vi "GUMSSequenceGeneratorV3.vi"() -> ()   [LabVIEW 2011]
uses:
  Kelvinox drivers/ITCAPPS - Copie.LLB/ITCSignal.ctl
  Kelvinox drivers/ITCAPPS.LLB/ITCSignals.ctl
  DAC/Visa name1.vi
  GlobalVar.vi
  stopButton.vi
  monochromatorcontrol/perHandlemonochromator.vi
  monochromatorcontrol/libPhyspec.lvlib
panel:
  out "loopchange 2":u32
  out "LockinX":string[][](array[string])
  in  "Device Cluster":T3={"K2400 1"="", "K2400_1"=FALSE, "K2400 2"="", "K2400_2"=FALSE, "TIC"="", "Tcontrol"="OFF", "DAC"="", "DAC present"=FALSE, "Bfield query"=FALSE, "Wvlen query"=FALSE, "ITC signal"={"ITC"=0, "Signal"=enum."Sensor 1"}, "DMMX"=[["DMM1", ""]], "LockinX"=[["DMM1", ""]]}
  in  "Gain Cluster":T4={"Vsd"="Gate", "I 2probe"="Gate", "Vxy"="Gate", "Vxx"="Gate", "I leak BG"="Gate", "I leak TG"="Gate", "I Gain 1"=1000000.0, "V Gain 1"=1.0, "conversion factor BG"=1.0, "Vin / Vout 1"=1.0, "V Gain 2"=1.0, "Vin / Vout 2"=1.0, "V Gain 3"=1.0, "Vin / Vout 3"=1.0, "I Gain 2"=1000000.0, "I Gain 3"=1000000.0, "V BG"="Gate", "V TG"="Gate", "conversion factor TG"=1.0, "Vin / Vout 4"=1.0, "Vin / Vout 5"=1.0, "Manual Gain 1"=1.0, "Manual Gain 2"=1.0, "Manual Gain 3"=1.0, "V / I 4"="Gate", "V / I 3"="Gate", "Gain V/I3"=1.0, "Gain V/I4"=1.0} {"conversion factor TG" items=["1 V/V"=1.0, "4 V/V"=4.0, "15 V/V"=15.0, "30 V/V"=30.0, "45 V/V"=45.0]; "I Gain 3" items=["1"=1.0, "10"=10.0, "100"=100.0, "1K"=1000.0, "10K"=10000.0, "100K"=100000.0, "1M"=1000000.0, "10M"=10000000.0, "100M"=100000000.0, "1G"=1000000000.0]; "I Gain 2" items=["1"=1.0, "10"=10.0, "100"=100.0, "1K"=1000.0, "10K"=10000.0, "100K"=100000.0, "1M"=1000000.0, "10M"=10000000.0, "100M"=100000000.0, "1G"=1000000000.0]; "V Gain 3" items=["1"=1.0, "10"=10.0, "100"=100.0, "1K"=1000.0, "10K"=10000.0]; "V Gain 2" items=["1"=1.0, "10"=10.0, "100"=100.0, "1K"=1000.0, "10K"=10000.0]; "conversion factor BG" items=["1 V/V"=1.0, "4 V/V"=4.0, "15 V/V"=15.0, "30 V/V"=30.0, "45 V/V"=45.0]; "V Gain 1" items=["1"=1.0, "10"=10.0, "100"=100.0, "1K"=1000.0, "10K"=10000.0]; "I Gain 1" items=["1"=1.0, "10"=10.0, "100"=100.0, "1K"=1000.0, "10K"=10000.0, "100K"=100000.0, "1M"=1000000.0, "10M"=10000000.0, "100M"=100000000.0, "1G"=1000000000.0]}
  out "counter 2":i32
  out "DMMX":string[][](array[string])
  out "Bloop gen":u32
  out "WVlenloop gen":u32
  out "Tloop gen":u32
  out "loopchange":u32
  out "DACindic":bool
  in  "EmptyAllArrays":bool
  in  "Sweep back to zero":bool
  out "counter":i32
  out "Num elements in col":i32[](array[numeric])
  out "Current col":i32
  in  "Refresh Rate [ms]":i32=1000 min=0
  out "Current sweep":dbl
  out "ITC ref":T1={"ITC"=0, "Signal"=enum."Sensor 3"}
  in  "Cancel run":bool
  out "DAC":refnum<visa-resource-name>
  out "K2400 2":refnum<visa-resource-name>
  out "Lockin1":refnum<visa-resource-name>
  out "K2400 1":refnum<visa-resource-name>
  out "Total sweep sequence":dbl[][](array[numeric])
  in  "Tab Control":T5(tab)
  in  "Sweep Toothsaw":bool
  in  "Loop Cluster":T6
  in  "START":bool
  in  "genTotalSequence":bool
  out "row state":i32[](array[numeric])
  out "Priority type array":string[](array[string])
  out "TotalPnts":dbl
  in  "Sweep back\nto zero?":bool
  in  "Conversion Factor Fix\n1 V = ??":dbl=1.0
  in  "Fix type":string(combo)
  in  "Sweep Bias":dbl[](array[numeric])
  in  "Fix Bias":dbl[](array[numeric])
  in  "Priority sweep":i32=2
  in  "Priority fix":i32=2
  in  "sweep start [V]":dbl=-1.0 min=-200.0 max=200.0
  in  "sweep stop [V]":dbl=-5.0 min=-250.0 max=250.0
  in  "Nb steps":i32=800
  in  "sweep stop 2 [V]":dbl min=-250.0 max=250.0
  in  "Nb steps 2":i32
  in  "Nb Sweep":i32=1
  in  "Nb steps fix2":i32
  in  "Fix stop 2":dbl min=-250.0 max=250.0
  in  "Nb steps fix":i32=800
  in  "Fix stop":dbl=-5.0 min=-250.0 max=250.0
  in  "Fix start":dbl=-1.0 min=-200.0 max=200.0
  in  "genSweepArray":bool
  in  "genFixArray":bool
  in  "Sweep Instrument":string(combo)
  in  "Conversion Factor Sweep\n1 V = ??":dbl=1.0
  in  "Fix Instrument":string(combo)
  in  "Sweep type":string(combo)
  in  "V step K2400 [V]":dbl=0.001
  in  "genSweepArray sweeploop":bool
  in  "genfixArray fixlooop simple":bool
  in  "Nb steps VI4 2":i32
  in  "VI4 stop2":dbl min=-250.0 max=250.0
  in  "Nb steps VI4":i32=800
  in  "VI4 stop1":dbl=-5.0 min=-250.0 max=250.0
  in  "genVI4Array":bool
  in  "genVI4Array simple":bool
  in  "Increase neg":dbl
  in  "Steps neg":dbl
  in  "Sweeps":i32
  in  "Steps 2":dbl
  in  "Bgstop 2":dbl
  in  "Steps":dbl
  in  "Bgstop":dbl
  in  "IOL ramp":dbl[](array[numeric])
  in  "VI 4 Array":dbl[](array[numeric])
  in  "Bgstart":dbl
  in  "Loops":i32
  in  "Increase pos":dbl
  in  "Steps pos":dbl
  in  "genIonicRamp":bool
  in  "Conversion Factor IOL Ramp\n1 V = ??":dbl=1.0
  in  "Conversion Factor VI4\n1 V = ??":dbl=1.0
  in  "VI4 start (V or I)":dbl=-1.0 min=-200.0 max=200.0
  in  "Stabilization Time (s)":i32 min=-200 max=200
  in  "T Rate [K/min]":dbl min=-200.0 max=200.0
  in  "T [K]":dbl[](array[numeric])
  in  "Priority T":i32=2
  in  "Nb T steps":i32=800
  in  "T stop [K]":dbl=-1.0 min=-200.0 max=200.0
  in  "T start [K]":dbl=-1.0 min=-200.0 max=200.0
  in  "genTarray":bool
  in  "Add T points":bool
  in  "Zero ramp Rate [T/min] 2":dbl=0.2 min=-200.0 max=200.0
  in  "Sweep Field back to zero":bool
  in  "B [T]":dbl[](array[numeric])
  in  "B start [T]":dbl=-1.0 min=-200.0 max=200.0
  in  "B stop [T]":dbl=-1.0 min=-200.0 max=200.0
  in  "Sweep Rate [T/min]":dbl=0.1 min=-200.0 max=200.0
  in  "Nb B steps":i32=800
  in  "GenBarray":bool
  in  "Add B points":bool
  in  "Set Persistent":bool=TRUE
  in  "PEM retardation (lambda)":dbl=1.0 min=0.0 max=1.0
  in  "PEM present ?":bool=TRUE
  in  "Power stabilization":bool=TRUE
  in  "Wvlen Start [nm]":dbl=400.0
  in  "Wavelength [nm]":dbl[](array[numeric])
  in  "genWVLEN array":bool
  in  "Add wvlen points":bool
  in  "Nb Wvlen steps":i32=350
  in  "Wvlen stop [nm]":dbl=1100.0
  out "Laser Power [W]":dbl format="%#.2g"
  in  "PEM VISA":refnum<visa-resource-name>
  in  "START FC":bool
  out "Field ok !":bool
  in  "Bipolar":bool
  in  "High T (K)":dbl
  in  "Temperature Up rate (K/min)":dbl
  in  "Waiting time (min)":dbl
  in  "Base T (K)":dbl
  in  "sweep rate B (T/min)":dbl
  in  "Cooling field (T)":dbl
  out "I am":string
  in  "File Basename":string
  out "Bias factor":dbl
  in  "Nb steps Increase 2":dbl=10.0
  in  "Gate Increase 2 (V)":dbl=0.1
  in  "Nb steps Increase":dbl=10.0
  in  "Gate Increase (V)":dbl=-0.1
  out "x .or. y?":bool
  in  "Step Delay (ms)":dbl=1000.0
  out "Total Progress":dbl(slide) scale=0.0..1.0
  in  "Nb Loop":i32
  out "Nb Loop Indicator":i32=2
  out "Nb Sweep Indicator":i32=3
  out "conversion factor sweep":dbl(ring)=1.0 items=["1 V/V"=1.0, "4 V/V"=4.0, "15 V/V"=15.0, "30 V/V"=30.0, "45 V/V"=45.0]
  in  "stop":bool
  in  "V step [V]":dbl=0.001
  in  "Folder Name":path=path "D:/users/marc/20180122_LiIon_EL/Freezing02/OutputHighT002p2.dat"
  # "Magnetic Field"
  # "Wavelength"
  # "IV Sweep Setting"
  # "IV Fix Setting"
  # "Ionic Liquid Ramp"
  # "VI 4 Array"
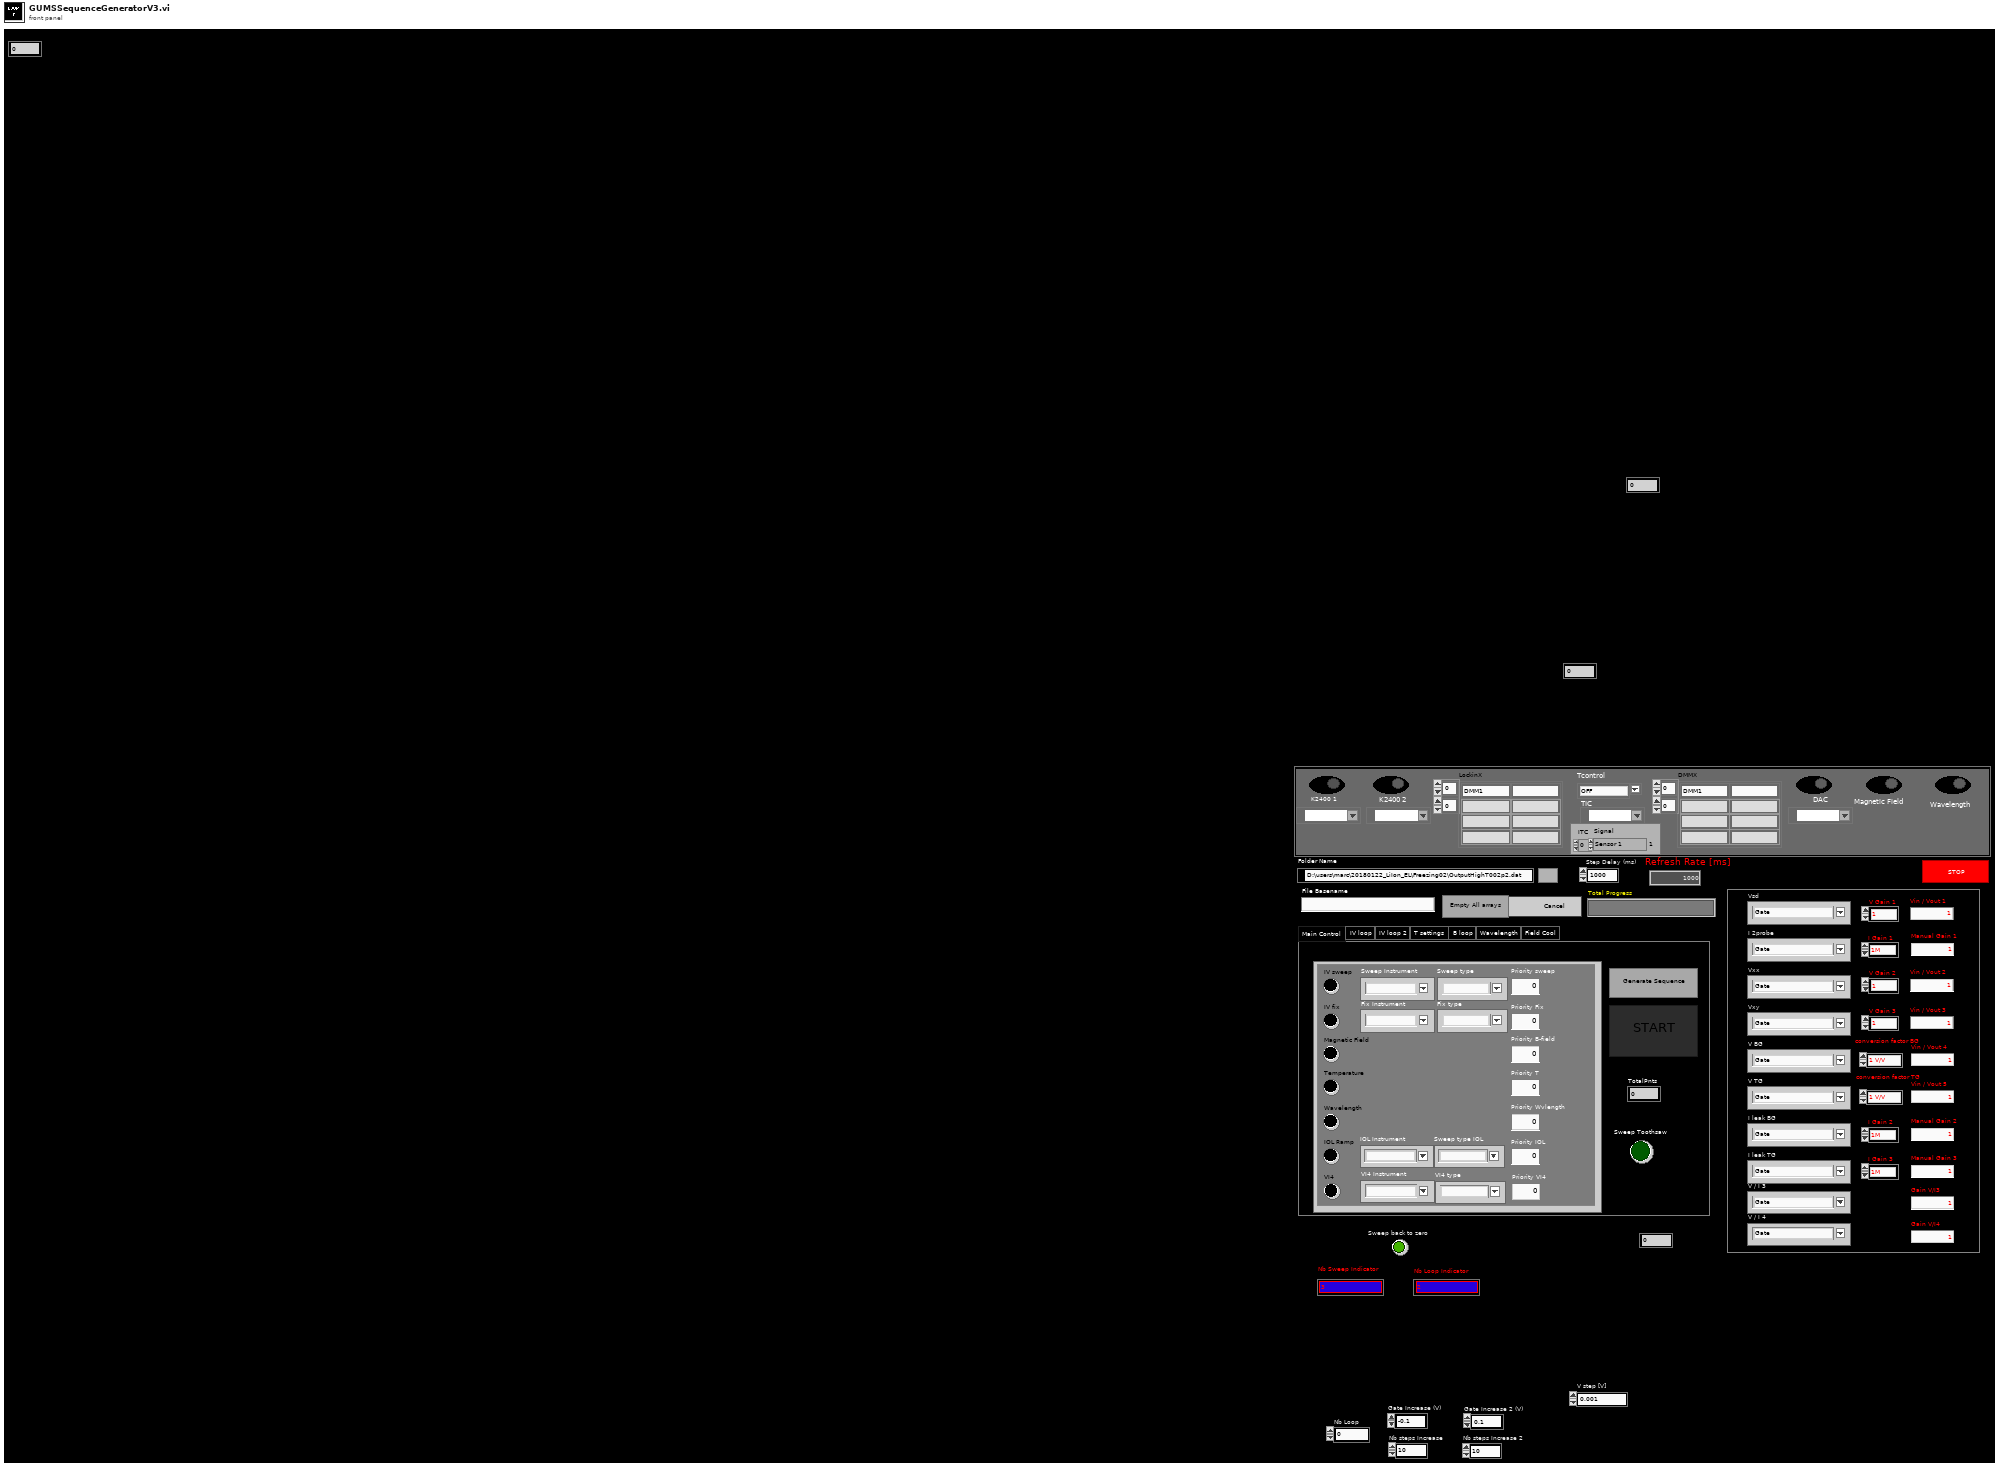
[diagram p1: front panel]
types:
  T1 = typedef "ITCSignal.ctl" = cluster{"ITC":u16, "Signal":T2}
  T2 = typedef "ITCSignals.ctl" = enum16{"Setpoint", "Sensor 1", "Sensor 2", "Sensor 3", "Needle Valve %", "Heater %"}
  T3 = cluster{"K2400 1":refnum<visa-resource-name>, "K2400_1":bool, "K2400 2":refnum<visa-resource-name>, "K2400_2":bool, "TIC":refnum<visa-resource-name>, "Tcontrol":string, "DAC":refnum<visa-resource-name>, "DAC present":bool, "Bfield query":bool, "Wvlen query":bool, "ITC signal":T1, "DMMX":string[][], "LockinX":string[][]}
  T4 = cluster{"Vsd":string, "I 2probe":string, "Vxy":string, "Vxx":string, "I leak BG":string, "I leak TG":string, "I Gain 1":dbl, "V Gain 1":dbl, "conversion factor BG":dbl, "Vin / Vout 1":dbl, "V Gain 2":dbl, "Vin / Vout 2":dbl, "V Gain 3":dbl, "Vin / Vout 3":dbl, "I Gain 2":dbl, "I Gain 3":dbl, "V BG":string, "V TG":string, "conversion factor TG":dbl, "Vin / Vout 4":dbl, "Vin / Vout 5":dbl, "Manual Gain 1":dbl, "Manual Gain 2":dbl, "Manual Gain 3":dbl, "V / I 4":string, "V / I 3":string, "Gain V/I3":dbl, "Gain V/I4":dbl}
  T5 = enum32{"Main Control", "IV loop", "IV loop 2", "T settings", "B loop", "Wavelength", "Field Cool"}
  T6 = cluster{"Sweep Instrument":string, "Sweep type":string, "Fix Instrument":string, "Fix type":string, "IV sweep":bool, "IV fix":bool, "Magnetic Field":bool, "Temperature":bool, "Wavelength":bool, "Priority sweep":dbl, "Priority Fix":dbl, "Priority B-field":dbl, "Priority T":dbl, "Priority Wvlength":dbl, "IOL Instrument":string, "Sweep type IOL":string, "IOL Ramp":bool, "Priority IOL":dbl, "VI4 Instrument":string, "VI4 type":string, "VI4":bool, "Priority VI4":dbl}
  T7 = cluster{"Power Stabilization":bool, "Laser Power [W]":dbl, "Power precision":dbl}
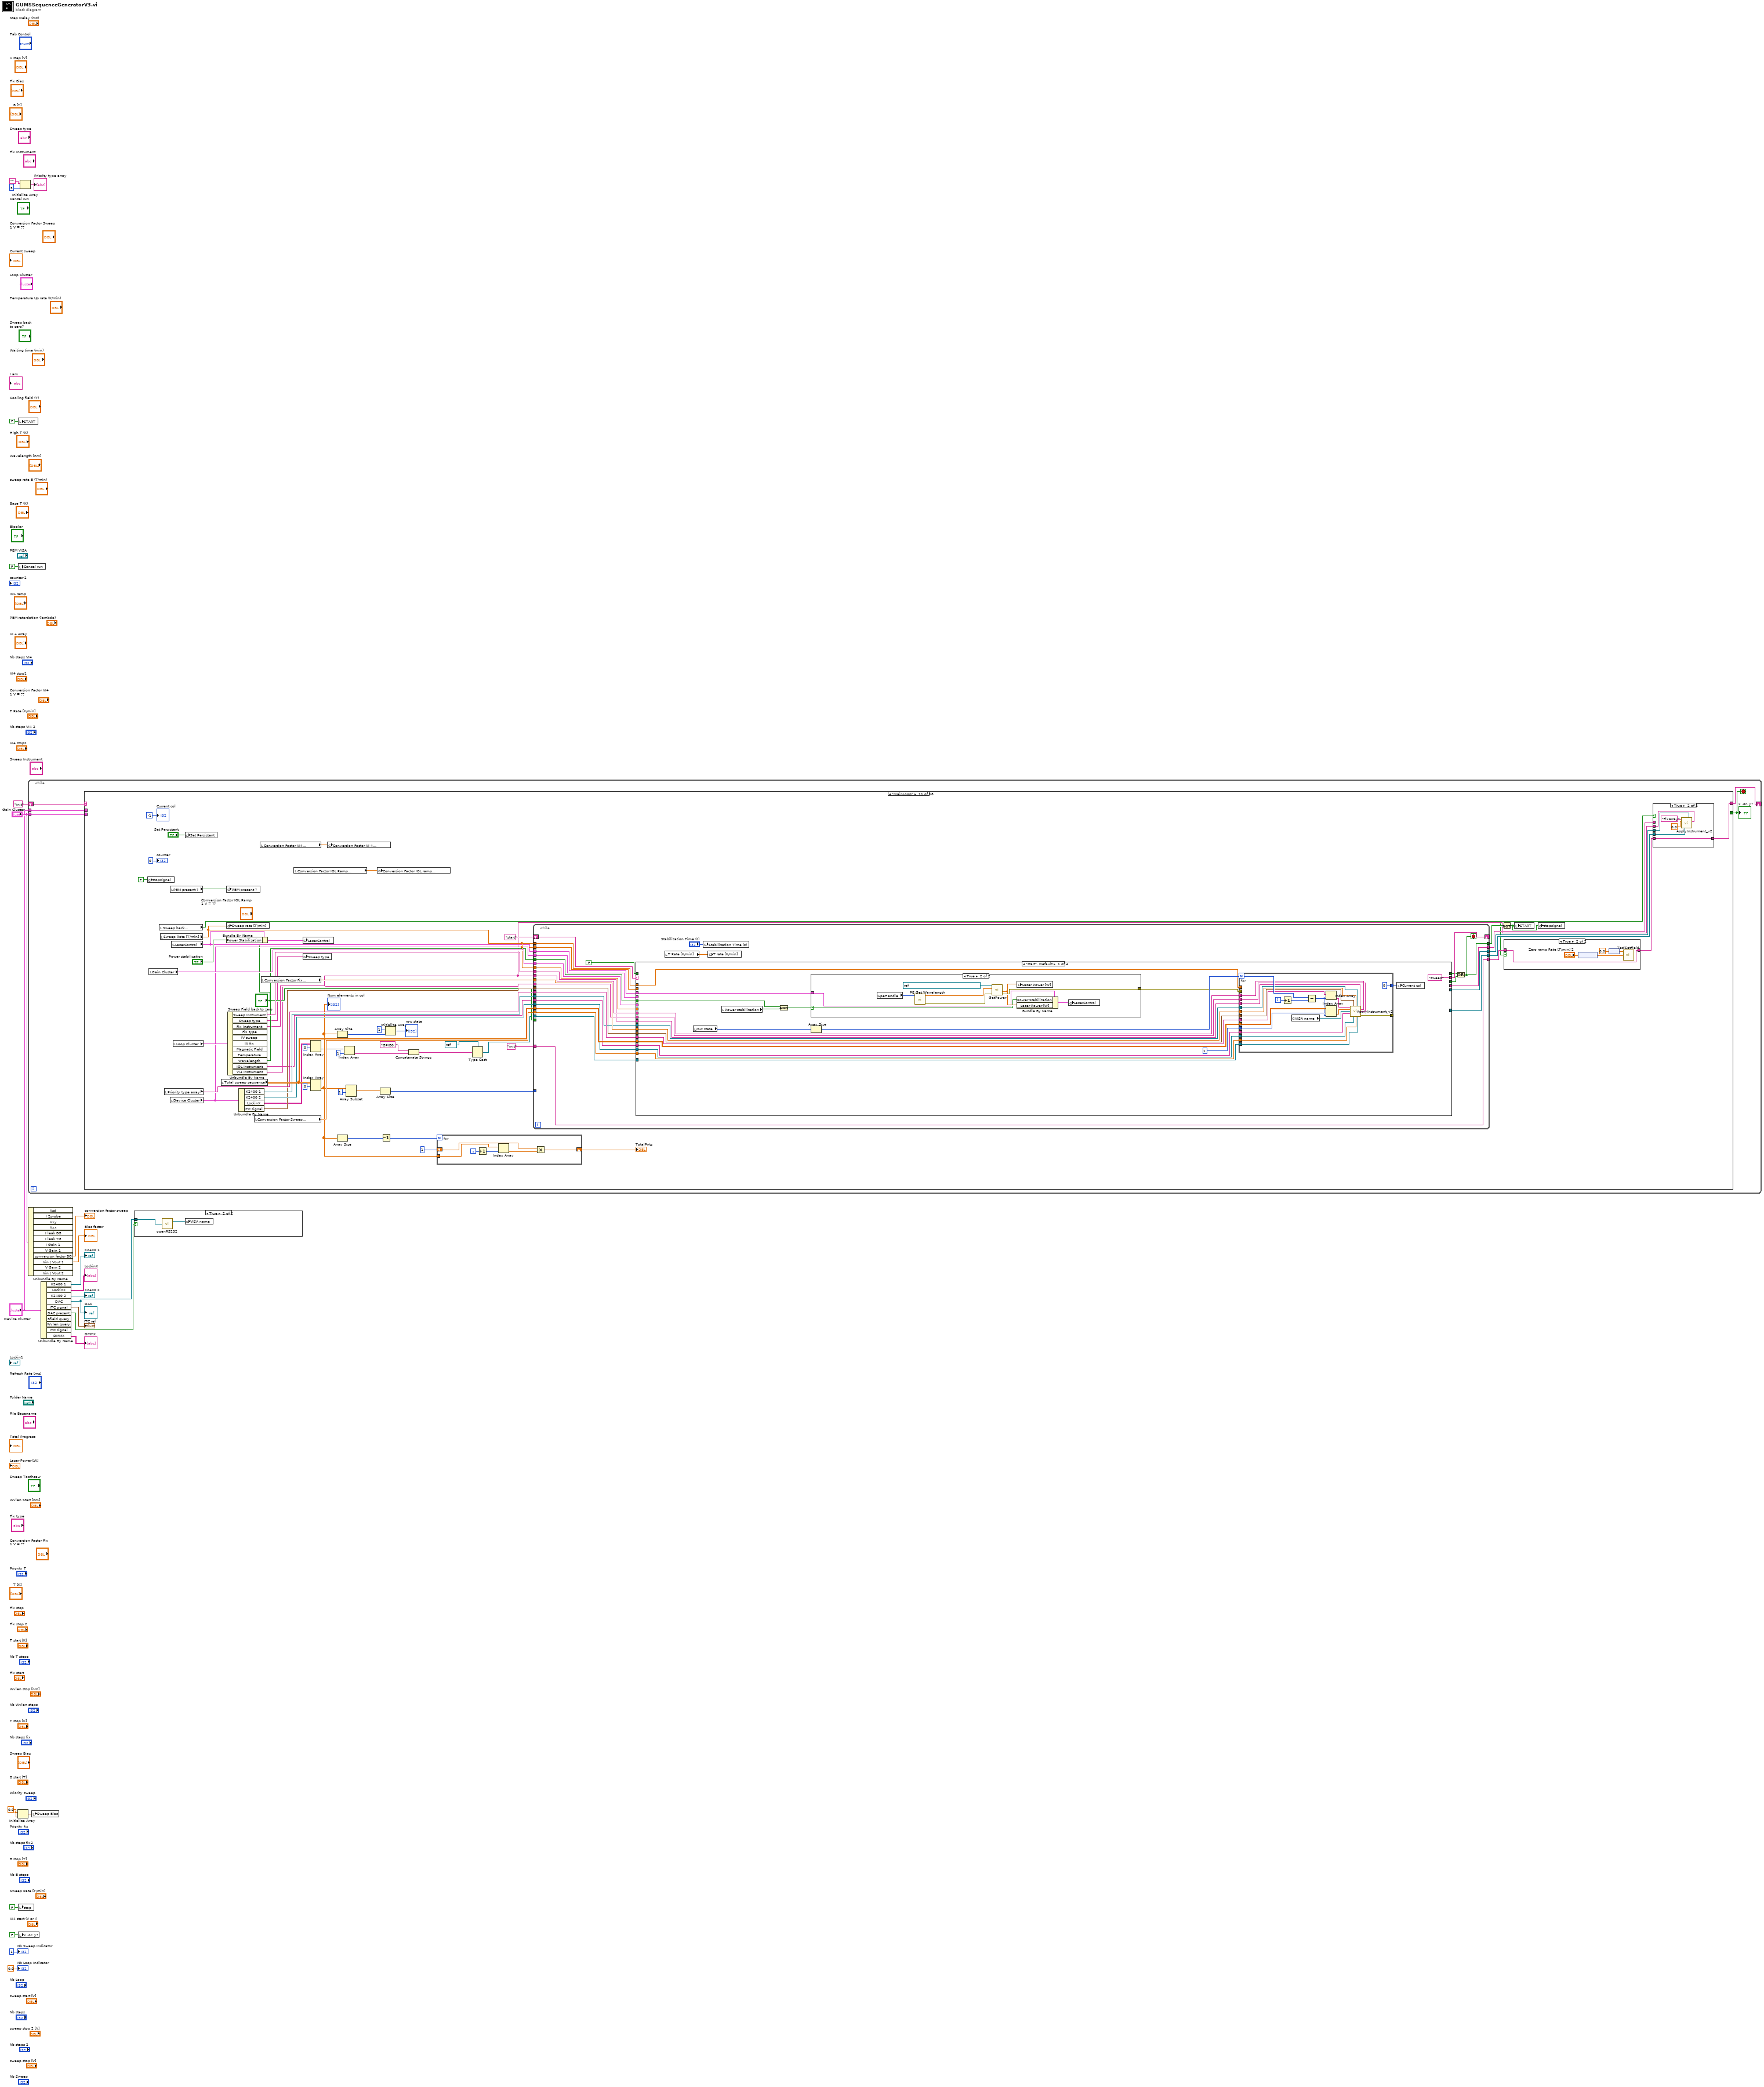
[diagram p0: block diagram]
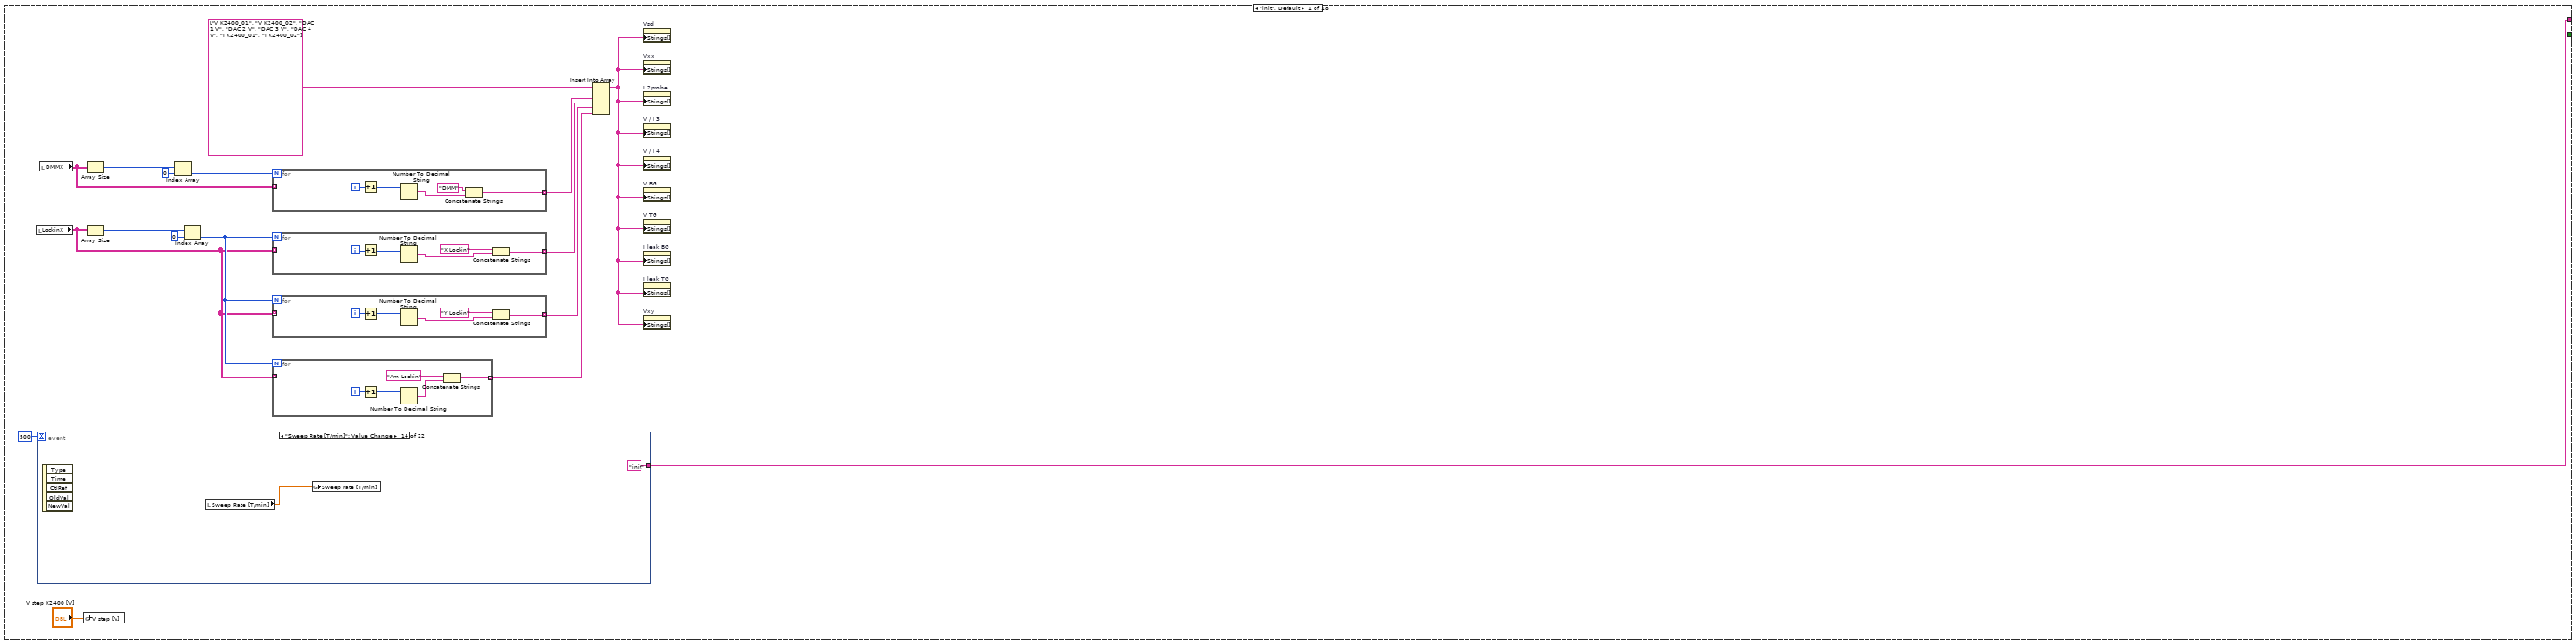
[diagram p3: hidden frame]
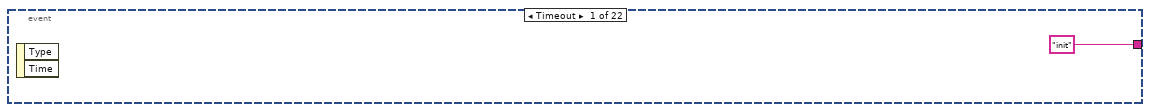
[diagram p4: hidden frame]
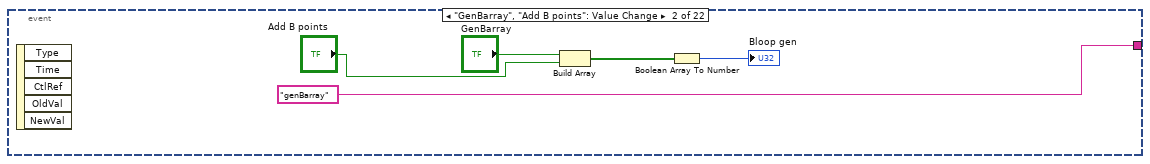
[diagram p5: hidden frame]
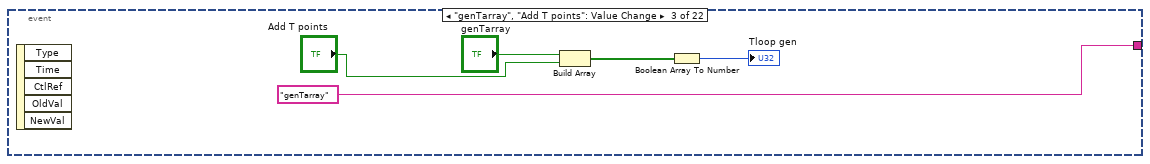
[diagram p6: hidden frame]
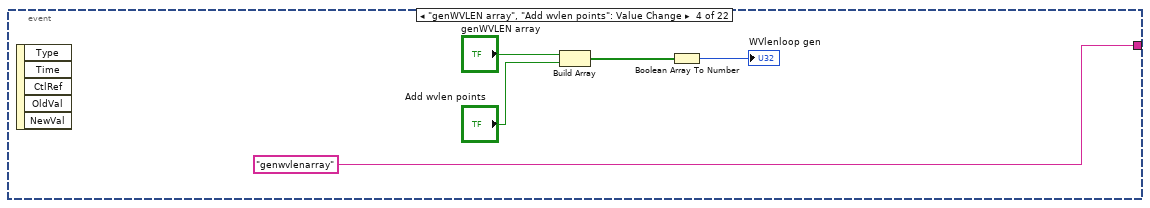
[diagram p7: hidden frame]
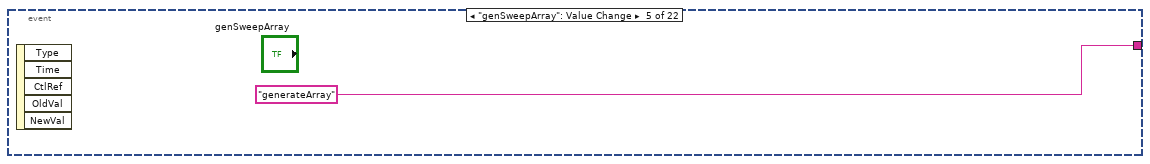
[diagram p8: hidden frame]
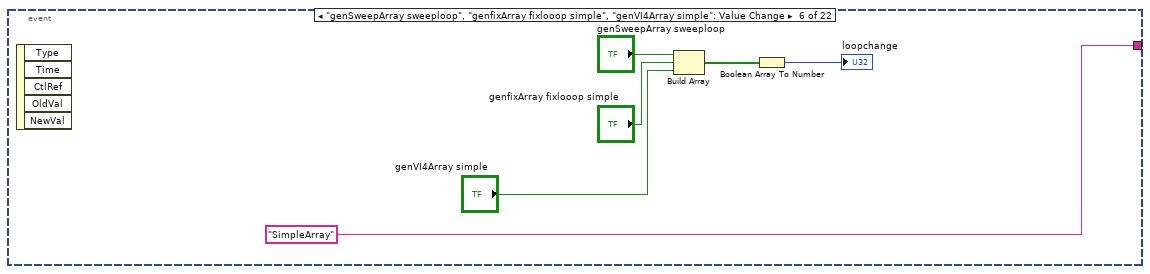
[diagram p9: hidden frame]
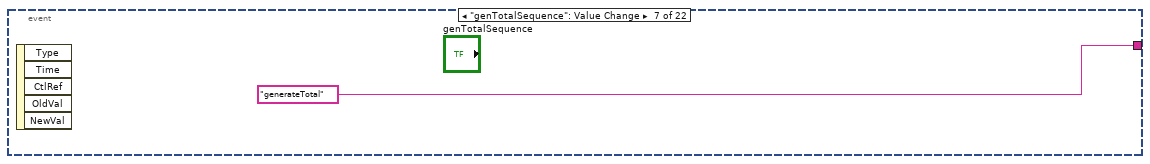
[diagram p10: hidden frame]
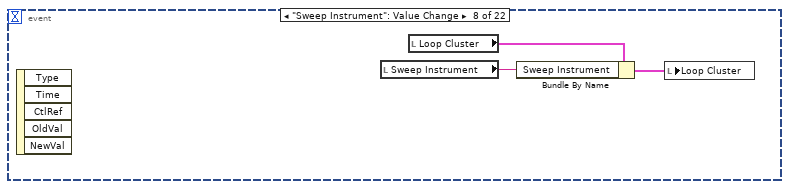
[diagram p11: hidden frame]
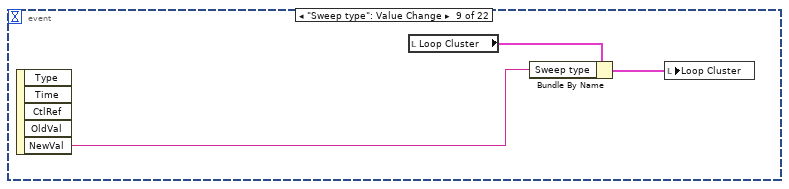
[diagram p12: hidden frame]
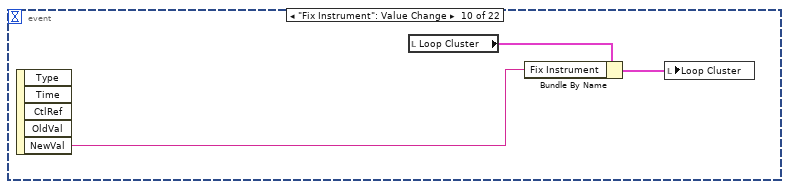
[diagram p13: hidden frame]
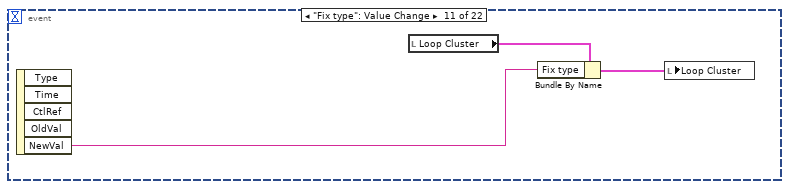
[diagram p14: hidden frame]
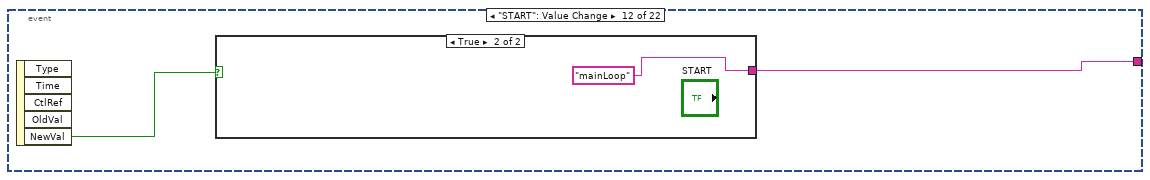
[diagram p15: hidden frame]
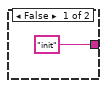
[diagram p16: hidden frame]
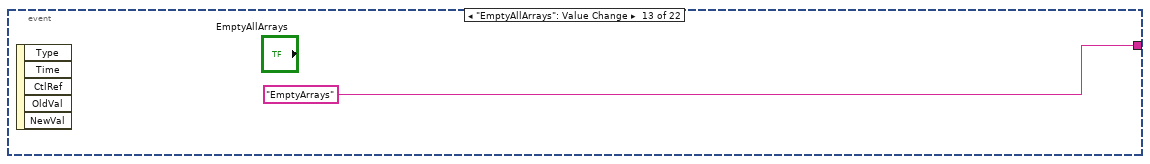
[diagram p17: hidden frame]
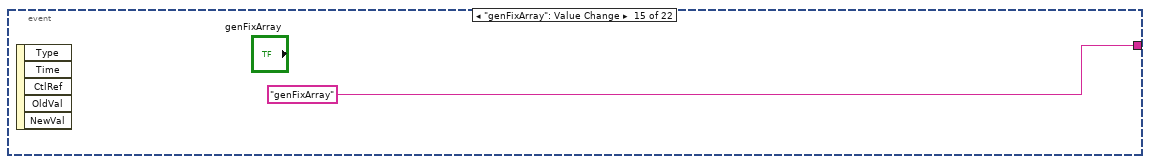
[diagram p18: hidden frame]
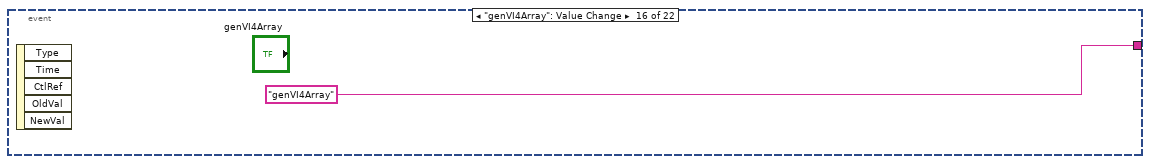
[diagram p19: hidden frame]
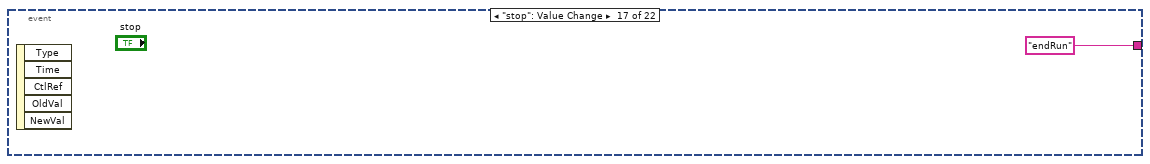
[diagram p20: hidden frame]
diagram:
  w8 = 0.0
  n1 = Initialize Array(w8, w8) -> (w9:dbl[])
  n2 = local write "START"(FALSE ("START")) -> ()
  n3 = local write "Cancel run"(FALSE ("Cancel run")) -> ()
  n4 = local write "stop"(FALSE ("stop")) -> ()
  n5 = local write "x .or. y?"(FALSE ("x .or. y?")) -> ()
  n6 = Initialize Array("", 5 ("dimension size")) -> (→"Priority type array":string[])
  n7 = while {
    shift-right: [w24] -> _
    shift-left: "init" -> [w28]
    tunnel: "Gain Cluster" -> [w26]
    tunnel: "Device Cluster" -> [w25]
    stop <- w27 stop-if-true
    n8 = case shown="\"mainLoop\"" w28 {
      tunnel: [_ _ _ _ _ _ _ _ _ _ _ _ TRUE _ _ _ _ _] -> w27
      tunnel: [w44 "init" "init" "init" "init" "init" "init" "init" "init" "init" w346 "generateArray" "" "init" w659 w668 "init" "init"] -> w24
      tunnel: w26 -> [_ _ _ _ _ _ _ _ _ _ _ _ _ _ _ _ _ _]
      tunnel: w25 -> [_ _ _ _ _ _ _ _ _ _ _ _ _ _ _ _ _ _]
      frame "init", Default {
        n9 = local read "LockinX"() -> (w33:string[][])
        n10 = event shown="[13] \"Sweep Rate [T/min]\": Value Change" {
          selector: _ -> [_ _ _ _ _ _ _ _ _ _ _ _ _ _ _ _ _ _ _ _ _ _]
          dyn-events: _ -> [_ _ _ _ _ _ _ _ _ _ _ _ _ _ _ _ _ _ _ _ _ _]
          timeout: 500 -> [_ _ _ _ _ _ _ _ _ _ _ _ _ _ _ _ _ _ _ _ _ _]
          tunnel: ["init" "genBarray" "genTarray" "genwvlenarray" "generateArray" "SimpleArray" "generateTotal" _ _ _ _ w102 "EmptyArrays" "init" "genFixArray" "genVI4Array" "endRun" "DACioload" "PEMinit" "IOLramp" "setRetard" "FCprocedure"] -> w44
          event Timeout {
            n11 = event-data() -> ()  [unwired: 1 in, 2 out]
          }
          event "GenBarray", "Add B points": Value Change {
            n12 = event-data() -> ()  [unwired: 1 in, 5 out]
            n13 = Build Array("GenBarray", "Add B points") -> (w70:bool[])
            n14 = Boolean Array To Number(Boolean array=w70) -> (number=→"Bloop gen":u32)
          }
          event "genTarray", "Add T points": Value Change {
            n15 = event-data() -> ()  [unwired: 1 in, 5 out]
            n16 = Build Array("genTarray", "Add T points") -> (w75:bool[])
            n17 = Boolean Array To Number(Boolean array=w75) -> (number=→"Tloop gen":u32)
          }
          event "genWVLEN array", "Add wvlen points": Value Change {
            n18 = event-data() -> ()  [unwired: 1 in, 5 out]
            n19 = Build Array("genWVLEN array", "Add wvlen points") -> (w80:bool[])
            n20 = Boolean Array To Number(Boolean array=w80) -> (number=→"WVlenloop gen":u32)
          }
          event "genSweepArray": Value Change {
            n21 = event-data() -> ()  [unwired: 1 in, 5 out]
          }
          event "genSweepArray sweeploop", "genfixArray fixlooop simple", "genVI4Array simple": Value Change {
            n22 = event-data() -> ()  [unwired: 1 in, 5 out]
            n23 = Build Array("genSweepArray sweeploop", "genfixArray fixlooop simple", "genVI4Array simple") -> (w85:bool[])
            n24 = Boolean Array To Number(Boolean array=w85) -> (number=→"loopchange":u32)
          }
          event "genTotalSequence": Value Change {
            n25 = event-data() -> ()  [unwired: 1 in, 5 out]
          }
          event "Sweep Instrument": Value Change {
            n26 = event-data() -> ()  [unwired: 1 in, 5 out]
            n27 = local read "Sweep Instrument"() -> (w91:string)
            n28 = local read "Loop Cluster"() -> (w92:T6)
            n29 = Bundle By Name(cluster=w92, "Sweep Instrument"=w91) -> (w90:T6)
            n30 = local write "Loop Cluster"(w90) -> ()
          }
          event "Sweep type": Value Change {
            n31 = event-data() -> ("NewVal"=w93:string)  [unwired: 1 in, 4 out]
            n32 = local read "Loop Cluster"() -> (w95:T6)
            n33 = Bundle By Name(cluster=w95, "Sweep type"=w93) -> (w94:T6)
            n34 = local write "Loop Cluster"(w94) -> ()
          }
          event "Fix Instrument": Value Change {
            n35 = event-data() -> ("NewVal"=w96:string)  [unwired: 1 in, 4 out]
            n36 = local read "Loop Cluster"() -> (w97:T6)
            n37 = Bundle By Name(cluster=w97, "Fix Instrument"=w96) -> (w98:T6)
            n38 = local write "Loop Cluster"(w98) -> ()
          }
          event "Fix type": Value Change {
            n39 = event-data() -> ("NewVal"=w101:string)  [unwired: 1 in, 4 out]
            n40 = local read "Loop Cluster"() -> (w100:T6)
            n41 = Bundle By Name(cluster=w100, "Fix type"=w101) -> (w99:T6)
            n42 = local write "Loop Cluster"(w99) -> ()
          }
          event "START": Value Change {
            n43 = event-data() -> ("NewVal"=w103:bool)  [unwired: 1 in, 4 out]
            n44 = case shown="True" w103 {
              tunnel: ["init" "mainLoop"] -> w102
              frame False {
              }
              frame True {
              }
            }
          }
          event "EmptyAllArrays": Value Change {
            n45 = event-data() -> ()  [unwired: 1 in, 5 out]
          }
          event "Sweep Rate [T/min]": Value Change {
            n46 = event-data() -> ()  [unwired: 1 in, 5 out]
            n47 = local read "Sweep Rate [T/min]"() -> (w108:dbl)
            n48 = global write "GlobalVar.vi" "Sweep rate [T/min]"(w108) -> ()
          }
          event "genFixArray": Value Change {
            n49 = event-data() -> ()  [unwired: 1 in, 5 out]
          }
          event "genVI4Array": Value Change {
            n50 = event-data() -> ()  [unwired: 1 in, 5 out]
          }
          event "stop": Value Change {
            n51 = event-data() -> ()  [unwired: 1 in, 5 out]
          }
          event "Device Cluster.DAC present": Value Change {
            n52 = event-data() -> ("NewVal"=→"DACindic":bool)  [unwired: 1 in, 4 out]
          }
          event "PEM present ?": Value Change {
            n53 = event-data() -> ()  [unwired: 1 in, 5 out]
          }
          event "genIonicRamp": Value Change {
            n54 = event-data() -> ()  [unwired: 1 in, 5 out]
          }
          event "PEM retardation (lambda)": Value Change {
            n55 = event-data() -> ()  [unwired: 1 in, 5 out]
          }
          event "START FC": Value Change {
            n56 = event-data() -> ()  [unwired: 1 in, 5 out]
          }
        }
        n57 = local read "DMMX"() -> (w38:string[][])
        n58 = global write "GlobalVar.vi" "V step [V]"("V step K2400 [V]") -> ()
        n59 = Array Size(array=w38) -> (size(s)=w41:i32[])
        n60 = Array Size(array=w33) -> (size(s)=w36:i32[])
        n61 = Index Array(array=w41, index=0) -> (element=w40:i32)
        n62 = Index Array(array=w36, index=0) -> (element=w34:i32)
        n63 = for {
          N: w40 -> [_]
          tunnel: w38 -> [_] mode=indexing
          tunnel: [w61] -> w37 mode=indexing
          i -> [w64]
          n64 = Increment(x=w64) -> (x+1=w62:i32)
          n65 = Number To Decimal String(number=w62) -> (decimal integer string=w63:string)  [unwired: 1 in]
          n66 = Concatenate Strings("DMM", w63) -> (w61:string)
        }
        n67 = for {
          N: w34 -> [_]
          tunnel: w33 -> [_] mode=indexing
          tunnel: [w56] -> w32 mode=indexing
          i -> [w59]
          n68 = Increment(x=w59) -> (x+1=w57:i32)
          n69 = Number To Decimal String(number=w57) -> (decimal integer string=w58:string)  [unwired: 1 in]
          n70 = Concatenate Strings("X Lockin", w58) -> (w56:string)
        }
        n71 = for {
          N: w34 -> [_]
          tunnel: [w51] -> w31 mode=indexing
          tunnel: w33 -> [_] mode=indexing
          i -> [w54]
          n72 = Increment(x=w54) -> (x+1=w52:i32)
          n73 = Number To Decimal String(number=w52) -> (decimal integer string=w53:string)  [unwired: 1 in]
          n74 = Concatenate Strings("Y Lockin", w53) -> (w51:string)
        }
        n75 = for {
          N: w34 -> [_]
          tunnel: [w46] -> w30 mode=indexing
          tunnel: w33 -> [_] mode=indexing
          i -> [w49]
          n76 = Increment(x=w49) -> (x+1=w47:i32)
          n77 = Number To Decimal String(number=w47) -> (decimal integer string=w48:string)  [unwired: 1 in]
          n78 = Concatenate Strings("Am Lockin", w48) -> (w46:string)
        }
        n79 = Insert Into Array(array=string[] ["V K2400_01", "V K2400_02", "DAC 1 V", "DAC 2 V", "DAC 3 V", "DAC 4 V", "I K2400_01", "I K2400_02"] ("Strings []"), new element #1=w37, new element #2=w32, new element #3=w31, new element #4=w30) -> (w29:string[])  [unwired: 1 in]
        n80 = property on="Vsd" class="CmbBox"("Strings[]"=w29) -> ()  [unwired: 2 in, 2 out]
        n81 = property on="Vxx" class="CmbBox"("Strings[]"=w29) -> ()  [unwired: 2 in, 2 out]
        n82 = property on="I 2probe" class="CmbBox"("Strings[]"=w29) -> ()  [unwired: 2 in, 2 out]
        n83 = property on="V / I 3" class="CmbBox"("Strings[]"=w29) -> ()  [unwired: 2 in, 2 out]
        n84 = property on="V / I 4" class="CmbBox"("Strings[]"=w29) -> ()  [unwired: 2 in, 2 out]
        n85 = property on="V BG" class="CmbBox"("Strings[]"=w29) -> ()  [unwired: 2 in, 2 out]
        n86 = property on="V TG" class="CmbBox"("Strings[]"=w29) -> ()  [unwired: 2 in, 2 out]
        n87 = property on="I leak BG" class="CmbBox"("Strings[]"=w29) -> ()  [unwired: 2 in, 2 out]
        n88 = property on="I leak TG" class="CmbBox"("Strings[]"=w29) -> ()  [unwired: 2 in, 2 out]
        n89 = property on="Vxy" class="CmbBox"("Strings[]"=w29) -> ()  [unwired: 2 in, 2 out]
      }
      frame "SimpleArray" {
        n90 = local read "loopchange"() -> (w118:u32)
        "loopchange 2" <- w118
        n91 = case shown="4" w118 {
          frame 0, Default {
          }
          frame 1 {
            n92 = local read "Nb steps"() -> (w122:i32)
            n93 = local read "sweep start [V]"() -> (w120:dbl)
            n94 = local read "sweep stop [V]"() -> (w121:dbl)
            n95 = call "createSimpleArray.vi"("nbpoint1"=w122, "Bgstop"=w121, "Bgstart"=w120) -> ("Outarray"=w123:dbl[])
            n96 = local write "Sweep Bias"(w123) -> ()
          }
          frame 2 {
            n97 = local read "Nb steps fix"() -> (w124:i32)
            n98 = local read "Fix start"() -> (w126:dbl)
            n99 = local read "Fix stop"() -> (w125:dbl)
            n100 = call "createSimpleArray.vi"("nbpoint1"=w124, "Bgstop"=w125, "Bgstart"=w126) -> ("Outarray"=w127:dbl[])
            n101 = local write "Fix Bias"(w127) -> ()
          }
          frame 4 {
            n102 = local read "Nb steps VI4"() -> (w128:i32)
            n103 = local read "VI4 stop1"() -> (w129:dbl)
            n104 = local read "VI4 start (V or I)"() -> (w130:dbl)
            n105 = call "createSimpleArray.vi"("nbpoint1"=w128, "Bgstop"=w129, "Bgstart"=w130) -> ("Outarray"=w131:dbl[])
            n106 = local write "VI 4 Array"(w131) -> ()
          }
        }
      }
      frame "generateTotal" {
        n107 = local read "Loop Cluster"() -> (w146:T6)
        n108 = Unbundle By Name(w146) -> ("IV sweep"=w166:bool, "IV fix"=w165:bool, "Magnetic Field"=w164:bool, "Temperature"=w163:bool, "Wavelength"=w162:bool, "Priority sweep"=w157:dbl, "Priority Fix"=w156:dbl, "Priority B-field"=w155:dbl, "Priority T"=w154:dbl, "Priority Wvlength"=w149:dbl, "Priority IOL"=w136:dbl, "IOL Ramp"=w137:bool, "VI4"=w134:bool, "Priority VI4"=w133:dbl)
        n109 = Build Array(w166, w165, w164, w163, w162, w137, w134) -> (w160:bool[])
        n110 = Decrement(x=w157) -> (x-1=w150:dbl)
        n111 = Decrement(x=w156) -> (x-1=w151:dbl)
        n112 = Decrement(x=w155) -> (x-1=w152:dbl)
        n113 = Decrement(x=w154) -> (x-1=w153:dbl)
        n114 = Decrement(x=w149) -> (x-1=w148:dbl)
        n115 = Decrement(x=w136) -> (x-1=w135:dbl)
        n116 = Decrement(x=w133) -> (x-1=w132:dbl)
        n117 = Boolean To (0,1)(Boolean=w160) -> (0, 1=w161:i16[])
        n118 = Add Array Elements(numeric array=w161) -> (sum=w159:i16)
        n119 = for {
          N: w159 -> [_]
          shift-right: [w195] -> w141
          shift-left: dbl[][] [] ("Array In") -> [w196]
          tunnel: w153 -> [w192]
          tunnel: w152 -> [w193]
          tunnel: w151 -> [w194]
          tunnel: w150 -> [w188]
          tunnel: w148 -> [w189]
          shift-right: [w183] -> w145
          shift-left: string[] [] -> [w181]
          tunnel: w135 -> [w178]
          tunnel: w132 -> [w175]
          i -> [w174]
          n120 = Equal?(x=w188, y=w174) -> (x = y?=w187:bool)
          n121 = Equal?(x=w194, y=w174) -> (x = y?=w186:bool)
          n122 = Equal?(x=w193, y=w174) -> (x = y?=w185:bool)
          n123 = Equal?(x=w192, y=w174) -> (x = y?=w184:bool)
          n124 = Equal?(x=w189, y=w174) -> (x = y?=w179:bool)
          n125 = Equal?(x=w178, y=w174) -> (x = y?=w177:bool)
          n126 = Equal?(x=w175, y=w174) -> (x = y?=w176:bool)
          n127 = Build Array(w187, w186, w185, w184, w179, w177, w176) -> (w191:bool[])
          n128 = Boolean Array To Number(Boolean array=w191) -> (number=w190:u32)
          n129 = case shown="64" w190 {
            tunnel: [_ "sweeparray" "Fixarray" "Bfield" ("Fix Instrument") "Temperature" "wavelength" "IOLramp" "VI4array"] -> w182
            tunnel: [_ w198 w200 w201 w203 w205 w208 w210] -> w180
            frame 0, Default {
            }
            frame 1 {
              n130 = local read "Sweep Bias"() -> (w198:dbl[])
            }
            frame 2 {
              n131 = local read "Fix Bias"() -> (w200:dbl[])
            }
            frame 4 {
              n132 = local read "B [T]"() -> (w201:dbl[])
            }
            frame 8 {
              n133 = local read "T [K]"() -> (w203:dbl[])
            }
            frame 16 {
              n134 = local read "Wavelength [nm]"() -> (w205:dbl[])
            }
            frame 32 {
              n135 = local read "IOL ramp"() -> (w208:dbl[])
            }
            frame 64 {
              n136 = local read "VI 4 Array"() -> (w210:dbl[])
            }
          }
          n137 = call "generateFinalArray.vi"("new array"=w180, "Array In"=w196) -> ("Array out"=w195:dbl[][])
          n138 = Build Array (concatenate)(w181, w182) -> (w183:string[])
        }
        "Total sweep sequence" <- w141
        n139 = local write "Priority type array"(w145) -> ()
        n140 = Index Array(array=w141, index (row)=0) -> (element=w138:dbl[])  [unwired: 1 in]
        n141 = Array Size(array=w138) -> (size(s)=w140:i32)
        n142 = Decrement(x=w140) -> (x-1=w139:i32)
        n143 = for {
          N: w139 -> [_]
          tunnel: w138 -> [w171]
          shift-right: [w168] -> w144
          shift-left: 1 ("index") -> [w169]
          i -> [w173]
          n144 = Increment(x=w173) -> (x+1=w172:i32)
          n145 = Index Array(array=w171, index=w172) -> (element=w170:dbl)
          n146 = Multiply(x=w169, y=w170) -> (x*y=w168:dbl)
        }
        n147 = local write "TotalPnts"(w144) -> ()
      }
      frame "generateArray" {
        w212 = 0.0 ("element")
        n148 = local read "Nb Sweep"() -> (w219:i32)
        n149 = local read "Priority type array"() -> (w217:string[])
        n150 = local read "Priority sweep"() -> (w213:i32)
        n151 = Initialize Array(w212, w212) -> (w211:dbl[])
        n152 = for {
          N: w219 -> [_]
          shift-right: [w223] -> w218
          shift-left: w211 -> [w222]
          n153 = local read "Nb steps 2"() -> (w227:i32)
          n154 = local read "Nb steps"() -> (w228:i32)
          n155 = local read "sweep stop 2 [V]"() -> (w225:dbl)
          n156 = local read "sweep start [V]"() -> (w226:dbl)
          n157 = local read "sweep stop [V]"() -> (w224:dbl)
          n158 = call "createLoopArray.vi"("Bgstop"=w224, "Bgstop2"=w225, "nbpoint1"=w228, "nbpoint2"=w227, "Bgstart"=w226) -> ("Outarray"=w221:dbl[])
          n159 = Build Array (concatenate)(w222, w221) -> (w223:dbl[])
        }
        n160 = Decrement(x=w213) -> (x-1=w214:i32)
        n161 = Replace Array Subset(array=w217, new element="sweeparray" ("new element/subarray"), index=w214) -> (w216:string[])
        n162 = local write "Priority type array"(w216) -> ()
        n163 = local write "Sweep Bias"(w218) -> ()
      }
      frame "IOLramp" {
        n164 = call "createLoopArrayIOL.vi"("Bgstart"="Bgstart", "Step Increase pos"="Steps pos", "Increase pos"="Increase pos", "Bgstop"="Bgstop", "nbpoint1"="Steps", "Bgstop2"="Bgstop 2", "Sweeps"="Sweeps", "Nb loops"="Loops", "Step Increase neg"="Steps neg", "Increase neg"="Increase neg", "nbpoint2"="Steps 2") -> ("Outarray"=w240:dbl[])  [unwired: 4 in]
        n165 = local write "IOL ramp"(w240) -> ()
      }
      frame "genFixArray" {
        n166 = local read "Nb Sweep"() -> (w244:i32)
        n167 = local read "Fix Bias"() -> (w243:dbl[])
        n168 = for {
          N: w244 -> [_]
          shift-right: [w248] -> w242
          shift-left: w243 -> [w247]
          n169 = local read "Nb steps fix"() -> (w253:i32)
          n170 = local read "Fix stop 2"() -> (w250:dbl)
          n171 = local read "Fix start"() -> (w251:dbl)
          n172 = local read "Fix stop"() -> (w249:dbl)
          n173 = local read "Nb steps fix2"() -> (w252:i32)
          n174 = call "createLoopArray.vi"("Bgstop"=w249, "Bgstop2"=w250, "nbpoint1"=w253, "nbpoint2"=w252, "Bgstart"=w251) -> ("Outarray"=w246:dbl[])
          n175 = Build Array (concatenate)(w247, w246) -> (w248:dbl[])
        }
        n176 = local write "Fix Bias"(w242) -> ()
      }
      frame "genVI4Array" {
        n177 = local read "Nb Sweep"() -> (w256:i32)
        n178 = local read "VI 4 Array"() -> (w255:dbl[])
        n179 = for {
          N: w256 -> [_]
          shift-right: [w260] -> w254
          shift-left: w255 -> [w259]
          n180 = local read "Nb steps VI4"() -> (w265:i32)
          n181 = local read "VI4 stop1"() -> (w261:dbl)
          n182 = local read "VI4 stop2"() -> (w262:dbl)
          n183 = local read "VI4 start (V or I)"() -> (w263:dbl)
          n184 = local read "Nb steps VI4 2"() -> (w264:i32)
          n185 = call "createLoopArray.vi"("Bgstop"=w261, "Bgstop2"=w262, "nbpoint1"=w265, "nbpoint2"=w264, "Bgstart"=w263) -> ("Outarray"=w258:dbl[])
          n186 = Build Array (concatenate)(w259, w258) -> (w260:dbl[])
        }
        n187 = local write "VI 4 Array"(w254) -> ()
      }
      frame "genTarray" {
        n188 = local read "Nb T steps"() -> (w268:i32)
        n189 = local read "Tloop gen"() -> (w271:u32)
        n190 = local read "T start [K]"() -> (w270:dbl)
        n191 = local read "T stop [K]"() -> (w269:dbl)
        n192 = local read "T [K]"() -> (w267:dbl[])
        n193 = case shown="2" w271 {
          tunnel: w270 -> [_ w277 w283]
          tunnel: w269 -> [_ w276 w282]
          tunnel: w268 -> [_ w275 w281]
          tunnel: [w273 w274 w278] -> w266
          tunnel: w267 -> [w273 _ w280]
          frame 0, Default {
          }
          frame 1 {
            n194 = call "createSimpleArray.vi"("nbpoint1"=w275, "Bgstop"=w276, "Bgstart"=w277) -> ("Outarray"=w274:dbl[])
          }
          frame 2 {
            n195 = call "createSimpleArray.vi"("nbpoint1"=w281, "Bgstop"=w282, "Bgstart"=w283) -> ("Outarray"=w279:dbl[])
            n196 = Insert Into Array(array=w280, new element=w279) -> (w278:dbl[])  [unwired: 1 in]
          }
        }
        n197 = local write "T [K]"(w266) -> ()
      }
      frame "genBarray" {
        n198 = local read "Nb B steps"() -> (w286:i32)
        n199 = local read "Bloop gen"() -> (w289:u32)
        n200 = local read "B start [T]"() -> (w288:dbl)
        n201 = local read "B stop [T]"() -> (w287:dbl)
        n202 = local read "B [T]"() -> (w285:dbl[])
        n203 = case shown="2" w289 {
          tunnel: w288 -> [_ w295 w301]
          tunnel: w287 -> [_ w294 w300]
          tunnel: w286 -> [_ w293 w299]
          tunnel: [w291 w292 w296] -> w284
          tunnel: w285 -> [w291 _ w298]
          frame 0, Default {
          }
          frame 1 {
            n204 = call "createSimpleArray.vi"("nbpoint1"=w293, "Bgstop"=w294, "Bgstart"=w295) -> ("Outarray"=w292:dbl[])
          }
          frame 2 {
            n205 = call "createSimpleArray.vi"("nbpoint1"=w299, "Bgstop"=w300, "Bgstart"=w301) -> ("Outarray"=w297:dbl[])
            n206 = Insert Into Array(array=w298, new element=w297) -> (w296:dbl[])  [unwired: 1 in]
          }
        }
        n207 = local write "B [T]"(w284) -> ()
      }
      frame "genwvlenarray" {
        n208 = local read "Wavelength [nm]"() -> (w303:dbl[])
        n209 = local read "Wvlen Start [nm]"() -> (w306:dbl)
        n210 = local read "Wvlen stop [nm]"() -> (w305:dbl)
        n211 = local read "Nb Wvlen steps"() -> (w304:i32)
        n212 = local read "WVlenloop gen"() -> (w307:u32)
        n213 = case shown="2" w307 {
          tunnel: w306 -> [_ w313 w319]
          tunnel: w305 -> [_ w312 w318]
          tunnel: w304 -> [_ w311 w317]
          tunnel: [w309 w310 w314] -> w302
          tunnel: w303 -> [w309 _ w316]
          frame 0, Default {
          }
          frame 1 {
            n214 = call "createSimpleArray.vi"("nbpoint1"=w311, "Bgstop"=w312, "Bgstart"=w313) -> ("Outarray"=w310:dbl[])
          }
          frame 2 {
            n215 = call "createSimpleArray.vi"("nbpoint1"=w317, "Bgstop"=w318, "Bgstart"=w319) -> ("Outarray"=w315:dbl[])
            n216 = Insert Into Array(array=w316, new element=w315) -> (w314:dbl[])  [unwired: 1 in]
          }
        }
        n217 = local write "Wavelength [nm]"(w302) -> ()
      }
      frame "mainLoop" {
        n218 = global write "stopButton.vi" "stopsignal"(FALSE) -> ()
        n219 = local read "Gain Cluster"() -> (w367:T4)
        n220 = local read "Sweep back\nto zero?"() -> (w348:bool)
        n221 = local read "Sweep Rate [T/min]"() -> (w342:dbl)
        n222 = local read "Priority type array"() -> (w365:string[])
        n223 = local read "PEM present ?"() -> (w325:bool)
        n224 = local read "Device Cluster"() -> (w359:T3)
        n225 = global read "GlobalVar.vi" "LaserControl"() -> (w337:T7)
        n226 = local read "Loop Cluster"() -> (w368:T6)
        n227 = global write "GlobalVar.vi" "Set Persistent"("Set Persistent") -> ()
        n228 = local read "Total sweep sequence"() -> (w369:dbl[][])
        n229 = global write "GlobalVar.vi" "PEM present ?"(w325) -> ()
        n230 = global write "GlobalVar.vi" "Sweep rate [T/min]"(w342) -> ()
        n231 = Bundle By Name(cluster=w337, "Power Stabilization"="Power stabilization") -> (w339:T7)
        n232 = Unbundle By Name(w368) -> ("Sweep Instrument"=w362:string, "Sweep type"=w324:string, "Fix Instrument"=w336:string, "Wavelength"=w338:bool, "IOL Instrument"=w321:string, "VI4 Instrument"=w320:string)  [unwired: 5 out]
        n233 = Unbundle By Name(w359) -> ("K2400 1"=w358:refnum<visa-resource-name>, "K2400 2"=w357:refnum<visa-resource-name>, "LockinX"=w330:string[][], "ITC signal"=w356:T1)
        n234 = local read "Conversion Factor Sweep\n1 V = ??"() -> (w361:dbl)
        n235 = local read "Conversion Factor VI4\n1 V = ??"() -> (w322:dbl)
        n236 = local read "Conversion Factor Fix\n1 V = ??"() -> (w360:dbl)
        n237 = local read "Conversion Factor IOL Ramp\n1 V = ??"() -> (w323:dbl)
        n238 = global write "GlobalVar.vi" "LaserControl"(w339) -> ()
        n239 = global write "GlobalVar.vi" "Sweep type"(w324) -> ()
        n240 = Index Array(array=w330, index (row)=0) -> (element=w327:string[])  [unwired: 1 in]
        n241 = Index Array(array=w369, index (row)=0) -> (element=w353:dbl[])  [unwired: 1 in]
        "Num elements in col" <- w353
        n242 = global write "GlobalVar.vi" "Conversion Factor VI 4\n1 V = ??"(w322) -> ()
        n243 = Array Size(array=w353) -> (size(s)=w374:i32)
        n244 = Array Size(array=w353) -> (size(s)=w355:i32)
        n245 = Index Array(array=w327, index=1) -> (element=w332:string)
        n246 = Array Subset(array=w353, index=1) -> (w372:dbl[])  [unwired: 1 in]
        n247 = global write "GlobalVar.vi" "Conversion Factor IOL ramp\n1 V = ??"(w323) -> ()
        n248 = Array Size(array=w372) -> (size(s)=w376:i32)
        n249 = Decrement(x=w355) -> (x-1=w354:i32)
        n250 = Initialize Array(1, w374) -> (→"row state":i32[])
        n251 = Concatenate Strings("GPIB0::" ("string"), w332) -> (w331:string)
        n252 = for {
          N: w354 -> [_]
          tunnel: w353 -> [w396]
          shift-right: [w393] -> w351
          shift-left: 1 ("index") -> [w394]
          i -> [w398]
          n253 = Increment(x=w398) -> (x+1=w397:i32)
          n254 = Index Array(array=w396, index=w397) -> (element=w395:dbl)
          n255 = Multiply(x=w394, y=w395) -> (x*y=w393:dbl)
        }
        "TotalPnts" <- w351
        n256 = Type Cast(type=refnum<visa-resource-name> refnum ("VISA resource name"), x=w331) -> (*(type *) &x=w326:refnum<visa-resource-name>)
        n257 = while {
          tunnel: w376 -> [_]
          shift-right: [w428] -> _
          shift-left: "start" -> [w429]
          tunnel: w369 -> [w427]
          tunnel: w367 -> [w426]
          tunnel: w359 -> [w425]
          tunnel: w365 -> [w424]
          tunnel: [w408] -> w364
          tunnel: "init" -> [w423]
          tunnel: [w423] -> w350
          tunnel: w336 -> [w422]
          tunnel: w362 -> [w421]
          tunnel: w342 -> [w420]
          tunnel: w342 -> [w419]
          tunnel: w342 -> [w418]
          tunnel: w361 -> [w417]
          tunnel: w360 -> [w416]
          tunnel: w358 -> [w415]
          tunnel: w357 -> [w414]
          tunnel: w326 -> [w413]
          tunnel: w356 -> [w412]
          tunnel: [w407] -> w345
          tunnel: [w406] -> w344
          tunnel: [w405] -> w343
          tunnel: w338 -> [w404]
          tunnel: w337 -> [w403]
          tunnel: "Sweep Field back to zero" -> [_]
          tunnel: w321 -> [w400]
          tunnel: w320 -> [w399]
          stop <- w408 stop-if-true
          n258 = case shown="\"start\", Default" w429 {
            selector: w429 -> [_ _ _ w630]
            tunnel: ["sweep" w523 w582 w630] -> w428
            tunnel: w427 -> [w448 w525 w578 _]
            tunnel: [_ _ _ TRUE] -> w410
            tunnel: w426 -> [_ w517 _ _]
            tunnel: w425 -> [_ w516 _ _]
            tunnel: w424 -> [w447 w511 w577 _]
            tunnel: w422 -> [w445 w508 w576 _]
            tunnel: w421 -> [w446 w507 w575 _]
            tunnel: w420 -> [_ _ w574 _]
            tunnel: w419 -> [w444 _ _ _]
            tunnel: w418 -> [_ _ _ _]
            tunnel: w417 -> [w443 w506 w572 _]
            tunnel: w416 -> [w442 w505 w573 _]
            tunnel: w415 -> [w439 w504 w568 _]
            tunnel: w414 -> [w440 w503 w569 _]
            tunnel: w413 -> [w438 w502 w570 _]
            tunnel: w412 -> [w441 w501 w571 _]
            tunnel: FALSE ("stopsignal") -> [_ w500 _ _]
            tunnel: [_ w496 _ _] -> w409
            tunnel: [_ w488 _ _] -> w407
            tunnel: [_ w487 _ _] -> w406
            tunnel: [_ w486 _ _] -> w405
            tunnel: w404 -> [w436 _ _ _]
            tunnel: w403 -> [w432 _ _ _]
            tunnel: w400 -> [w431 w485 w567 _]
            tunnel: w399 -> [w430 w484 w566 _]
            frame "start", Default {
              n259 = local read "row state"() -> (w451:i32[])
              n260 = local read "Power stabilization"() -> (w435:bool)
              n261 = And(x=w436, y=w435) -> (x .and. y?=w434:bool)
              n262 = case shown="True" w434 {
                selector: w434 -> [_ w453]
                tunnel: [_ w457] -> w433
                tunnel: w432 -> [_ w454]
                frame False {
                }
                frame True {
                  n263 = global read "perHandlemonochromator.vi" "peHandle"() -> (w461:u32)
                  n264 = call "PE Get Wavelength.vi"("peHandle"=w461) -> ("error out"=w458:errorcluster, "wavelength"=w460:dbl)  [unwired: 8 in, 1 out]
                  n265 = call "GetPower.vi"("error in (no error)"=w458, "Wavelength (nm)"=w460, "Input Device"=refnum<visa-resource-name> "USB0::0x1313::0x8072::P2007928::INSTR") -> ("error out"=w457:errorcluster, "Power (W)"=w456:dbl)  [unwired: 1 in, 2 out]
                  n266 = local write "Laser Power [W]"(w456) -> ()
                  n267 = Bundle By Name(cluster=w454, "Power Stabilization"=w453, "Laser Power [W]"=w456) -> (w455:T7)
                  n268 = global write "GlobalVar.vi" "LaserControl"(w455) -> ()
                }
              }
              n269 = Array Size(array=w451) -> (size(s)=w450:i32)
              n270 = for {
                N: w450 -> [w481]
                tunnel: 1 -> [w482]
                tunnel: w448 -> [w483]
                tunnel: w447 -> [w477]
                tunnel: w446 -> [w475]
                tunnel: w445 -> [w474]
                tunnel: w444 -> [_]
                tunnel: w443 -> [w473]
                tunnel: w442 -> [w472]
                tunnel: w441 -> [w471]
                tunnel: w440 -> [w470]
                tunnel: w439 -> [w469]
                tunnel: w438 -> [w468]
                tunnel: [w467] -> _
                tunnel: [0 ("Current col")] -> w437
                tunnel: w433 -> [_]
                tunnel: w431 -> [w464]
                tunnel: w430 -> [w462]
                i -> [w480]
                n271 = Increment(x=w480) -> (x+1=w479:i32)
                n272 = global read "Visa name1.vi" "VISA name"() -> (w463:refnum<visa-resource-name>)
                n273 = Subtract(x=w481, y=w479) -> (x-y=w476:i32)
                n274 = Index Array(array=w477, index=w476) -> (element=w465:string)
                n275 = Index Array(array=w483, index (row)=w482, index (col)=w476) -> (element=w478:dbl)
                n276 = call "ApplyInstrument_v2.vi"("Instrument"=w465, "ITC ref"=w471, "Conversion Factor Fix\n1 V = ??"=w472, "K2400 1"=w469, "Sweep Instrument"=w475, "Valin"=w478, "Fix Instrument"=w474, "DAC COM port"=w463, "VI4 Instrument"=w462, "IOL Instrument"=w464, "K2400 2"=w470, "Conversion Factor Sweep\n1 V = ??"=w473, "Lockin1"=w468) -> ("error out"=w467:errorcluster)  [unwired: 2 in]
              }
              n277 = local write "Current col"(w437) -> ()
            }
            frame "sweep" {
              w529 = 0 ("index")
              n278 = global write "stopButton.vi" "stopsignal"(w500) -> ()
              n279 = Index Array(array=w525, index (row)=w529, index (col)=w529) -> (element=w528:dbl)
              n280 = local read "Current col"() -> (w509:i32)
              n281 = local read "TotalPnts"() -> (w499:dbl)
              n282 = local read "row state"() -> (w522:i32[])
              n283 = local read "counter"() -> (w491:i32)
              n284 = local read "Refresh Rate [ms]"() -> (w497:i32)
              n285 = local read "Sweep Toothsaw"() -> (w489:bool)
              n286 = local read "File Basename"() -> (w514:string)
              n287 = local read "Folder Name"() -> (w515:path)
              n288 = Index Array(array=w522, index=w509) -> (element=w526:i32)
              n289 = Index Array(array=w511, index=w509) -> (element=w510:string)
              n290 = Increment(x=w491) -> (x+1=w495:i32)
              n291 = Quotient & Remainder(x=w491, y=2.0) -> (x-y*floor(x/y)=w493:dbl)  [unwired: 1 out]
              n292 = local write "counter"(w495) -> ()
              n293 = call "autoNameFile.vi"("num"=w491, "File Basename"=w514, "Folder Name"=w515) -> ("path"=w518:path)
              n294 = Not Equal To 0?(x=w493) -> (x != 0?=w490:bool)
              n295 = for {
                N: w528 -> [_]
                tunnel: [w557] -> w523
                tunnel: "changerow" -> [w557]
                tunnel: w509 -> [w545]
                tunnel: w525 -> [w546]
                tunnel: [w545] -> w520
                shift-right: [w556] -> _
                shift-left: w526 -> [w544]
                tunnel: [TRUE] -> w513
                tunnel: w510 -> [w539]
                tunnel: [w534] -> _
                tunnel: w508 -> [w536]
                tunnel: w507 -> [w553]
                tunnel: w506 -> [w552]
                tunnel: w505 -> [w551]
                tunnel: w504 -> [w538]
                tunnel: w503 -> [w537]
                tunnel: w502 -> [w550]
                tunnel: w501 -> [w549]
                tunnel: [w548] -> w496
                tunnel: [w547] -> _
                tunnel: w495 -> [w547]
                tunnel: [w547] -> w494
                tunnel: w490 -> [w543]
                tunnel: w489 -> [w540]
                tunnel: [w538] -> w488
                tunnel: [w537] -> w487
                tunnel: [w536] -> w486
                tunnel: w485 -> [w531]
                tunnel: w484 -> [w530]
                stop <- w548 stop-if-true
                n296 = And(x=w543, y=w540) -> (x .and. y?=w542:bool)
                n297 = Increment(x=w544) -> (x+1=w556:i32)
                n298 = global read "Visa name1.vi" "VISA name"() -> (w532:refnum<visa-resource-name>)
                n299 = local read "Cancel run"() -> (w548:bool)
                n300 = case shown="True" w542 {
                  tunnel: w544 -> [w558 w561]
                  tunnel: w546 -> [_ w565]
                  tunnel: w545 -> [_ w563]
                  tunnel: [w558 w560] -> w541
                  frame False {
                    # "forth"
                  }
                  frame True {
                    n301 = Decrement(x=w561) -> (x-1=w559:i32)
                    n302 = Index Array(array=w565, index (row)=0, index (col)=w563) -> (element=w562:dbl)
                    n303 = Subtract(x=w562, y=w559) -> (x-y=w560:dbl)
                  }
                }
                n304 = local read "Step Delay (ms)"() -> (w533:dbl)
                n305 = Index Array(array=w546, index (row)=w541, index (col)=w545) -> (element=w554:dbl)
                n306 = call "ApplyInstrument_v2.vi"("Instrument"=w539, "ITC ref"=w549, "Conversion Factor Fix\n1 V = ??"=w551, "K2400 1"=w538, "Sweep Instrument"=w553, "Valin"=w554, "Fix Instrument"=w536, "DAC COM port"=w532, "VI4 Instrument"=w530, "IOL Instrument"=w531, "K2400 2"=w537, "Conversion Factor Sweep\n1 V = ??"=w552, "Lockin1"=w550) -> ("error out"=w535:errorcluster)  [unwired: 2 in]
                n307 = call "wait.vi"("error in (no error)"=w535, "wait time (ms)"=w533) -> ("error in (no error) 2"=w534:errorcluster)
              }
              n308 = call "gums_measureLoopV3.vi"("File Name"=w518, "SaveDataQuery"=TRUE, "Gain Cluster 2"=w517, "Refresh Rate [ms]"=w497, "Device Cluster"=w516) -> ()  [unwired: 6 in]
              n309 = global write "stopButton.vi" "stopsignal"(w513) -> ()
              n310 = Divide(x=w494, y=w499) -> (x/y=w498:dbl)
              n311 = Increment(x=w520) -> (x+1=w524:i32)
              n312 = Replace Array Subset(array=w522, new element=1 ("new element/subarray"), index=w520) -> (w521:i32[])
              n313 = local write "row state"(w521) -> ()
              n314 = local write "Total Progress"(w498) -> ()
              n315 = local write "Current col"(w524) -> ()
            }
            frame "changerow" {
              n316 = local read "Current col"() -> (w579:i32)
              n317 = local read "row state"() -> (w589:i32[])
              n318 = Index Array(array=w589, index=w579) -> (element=w585:i32)
              n319 = local read "Num elements in col"() -> (w587:i32[])
              n320 = Increment(x=w585) -> (x+1=w584:i32)
              n321 = Index Array(array=w587, index=w579) -> (element=w592:i32)
              n322 = Array Size(array=w587) -> (size(s)=w586:i32)
              n323 = Greater?(x=w584, y=w592) -> (0:w591:bool)
              n324 = case shown="False" w591 {
                tunnel: [w618 0] -> w580
                tunnel: w584 -> [w618 _]
                tunnel: [w616 w624] -> w590
                tunnel: [w613 w621] -> w583
                tunnel: w579 -> [w617 w625]
                tunnel: w586 -> [_ w623]
                frame False {
                  n325 = Decrement(x=w617) -> (x-1=w616:i32)
                  n326 = Equal?(x=0, y=w616) -> (x = y?=w614:bool)
                  n327 = case shown="False" w614 {
                    tunnel: ["changerow" "sweep"] -> w613
                    frame False {
                    }
                    frame True {
                    }
                  }
                }
                frame True {
                  n328 = Increment(x=w625) -> (x+1=w624:i32)
                  n329 = Greater?(x=w624, y=w623) -> (0:w622:bool)
                  n330 = case shown="False" w622 {
                    tunnel: ["changerow" "stop"] -> w621
                    frame False {
                    }
                    frame True {
                    }
                  }
                }
              }
              n331 = local write "Current col"(w590) -> ()
              n332 = Replace Array Subset(array=w589, new element=w580, index=w579) -> (w588:i32[])
              n333 = Not Equal To 0?(x=w580) -> (x != 0?=w581:bool)
              n334 = local write "row state"(w588) -> ()
              n335 = case shown="True" w581 {
                tunnel: w583 -> [w593 w612]
                tunnel: [w593 w612] -> w582
                tunnel: w578 -> [_ w611]
                tunnel: w579 -> [_ w606]
                tunnel: w580 -> [_ w610]
                tunnel: w577 -> [_ w607]
                tunnel: w576 -> [_ w605]
                tunnel: w575 -> [_ w604]
                tunnel: w574 -> [_ _]
                tunnel: w573 -> [_ w603]
                tunnel: w572 -> [_ w602]
                tunnel: w571 -> [_ w601]
                tunnel: w570 -> [_ w600]
                tunnel: w569 -> [_ w599]
                tunnel: w568 -> [_ w598]
                tunnel: w567 -> [_ w596]
                tunnel: w566 -> [_ w594]
                frame False {
                }
                frame True {
                  n336 = Index Array(array=w611, index (row)=w610, index (col)=w606) -> (element=w608:dbl)
                  n337 = Index Array(array=w607, index=w606) -> (element=w597:string)
                  n338 = Wait (ms)(milliseconds to wait=u32 400) -> ()  [unwired: 1 out]
                  n339 = global read "Visa name1.vi" "VISA name"() -> (w595:refnum<visa-resource-name>)
                  n340 = call "ApplyInstrument_v2.vi"("Instrument"=w597, "ITC ref"=w601, "Conversion Factor Fix\n1 V = ??"=w603, "K2400 1"=w598, "Sweep Instrument"=w604, "Valin"=w608, "Fix Instrument"=w605, "DAC COM port"=w595, "VI4 Instrument"=w594, "IOL Instrument"=w596, "K2400 2"=w599, "Conversion Factor Sweep\n1 V = ??"=w602, "Lockin1"=w600) -> ()  [unwired: 2 in, 1 out]
                }
              }
            }
            frame "stop" {
            }
          }
          n341 = local read "T Rate [K/min]"() -> (w401:dbl)
          n342 = global write "GlobalVar.vi" "Stabilization Time (s)"("Stabilization Time (s)") -> ()
          n343 = global write "GlobalVar.vi" "T rate [K/min]"(w401) -> ()
          n344 = Or(x=w410, y=w409) -> (x .or. y?=w408:bool)
        }
        n345 = Not(x=w364) -> (.not. x?=w349:bool)
        n346 = case shown="True" "Sweep Field back to zero" {
          tunnel: w350 -> [w387 w392]
          tunnel: [w387 w392] -> w347
          frame False {
          }
          frame True {
            n347 = node("Zero ramp Rate [T/min] 2") -> (w391:dbl[unit])
            n348 = node(0.0) -> (w390:dbl[unit])
            n349 = call "TeslSetField.vi"("Sweep rate"=w391, "Field required:"=w390) -> ()  [unwired: 2 in, 2 out]
          }
        }
        n350 = local write "START"(w349) -> ()
        n351 = global write "stopButton.vi" "stopsignal"(w349) -> ()
        n352 = case shown="True" w348 {
          tunnel: w347 -> [w380 w386]
          tunnel: [w380 w386] -> w346
          tunnel: w345 -> [_ w383]
          tunnel: w344 -> [_ w382]
          tunnel: w343 -> [_ _]
          tunnel: w336 -> [_ w381]
          frame False {
          }
          frame True {
            n353 = call "ApplyInstrument_v2.vi"("Instrument"="Fixarray", "K2400 1"=w383, "Valin"=0.0, "Fix Instrument"=w381, "K2400 2"=w382) -> ()  [unwired: 10 in, 1 out]
          }
        }
        "Current col" <- -1 ("Current col")
        "counter" <- 0 ("counter")
      }
      frame "loopIncrease" {
        # "VERIFY IF THIS IS REALLY NECESSARY\n14.10.2020"
        n354 = local read "Nb steps 2"() -> (w638:i32)
        n355 = local read "Nb steps"() -> (w637:i32)
        n356 = local read "Nb Loop Indicator"() -> (w646:i32)
        n357 = local read "sweep stop 2 [V]"() -> (w639:dbl)
        n358 = local read "sweep stop [V]"() -> (w641:dbl)
        n359 = Add(x="Nb steps Increase 2", y=w638) -> (x+y=w634:dbl)
        n360 = Add(x=w639, y="Gate Increase 2 (V)") -> (x+y=w631:dbl)
        n361 = Add(x="Gate Increase (V)", y=w641) -> (x+y=w632:dbl)
        n362 = Add(x="Nb steps Increase", y=w637) -> (x+y=w633:dbl)
        n363 = Increment(x=w646) -> (x+1=w645:i32)
        n364 = local write "Nb Loop Indicator"(w645) -> ()
        n365 = local write "Nb steps 2"(w634) -> ()
        n366 = local write "sweep stop 2 [V]"(w631) -> ()
        n367 = local write "sweep stop [V]"(w632) -> ()
        n368 = local write "Nb steps"(w633) -> ()
        n369 = local write "Nb Sweep Indicator"(1 ("Nb Sweep Indicator")) -> ()
      }
      frame "endRun" {
        n370 = local read "Device Cluster"() -> (w649:T3)
        n371 = local read "PEM present ?"() -> (w647:bool)
        n372 = case shown="True" w647 {
          frame False {
          }
          frame True {
            n373 = local read "PEM VISA"() -> (w653:refnum<visa-resource-name>)
            n374 = call "HindsPEM100_VISASeriaClose.vi"("VISA session (for class)"=w653) -> ()  [unwired: 18 in, 1 out]
          }
        }
        n375 = case shown="True" "Sweep back to zero" {
          frame False {
          }
          frame True {
            n376 = call "K2400_ApplyVOLTsafe_GUMS.vi"("Voltage target [V]"=0.0) -> ()  [unwired: 2 in]
          }
        }
        n377 = Unbundle By Name(w649) -> ("DAC present"=w648:bool)
        n378 = case shown="True" w648 {
          frame False {
          }
          frame True {
            n379 = local read "DAC"() -> (w654:refnum<visa-resource-name>)
            n380 = call "closeRS232.vi"("VISA resource name"=w654) -> ()  [unwired: 2 in]
          }
        }
      }
      frame "EmptyArrays" {
        w657 = 0.0
        n381 = Initialize Array(w657, w657) -> (w656:dbl[])
        n382 = local write "B [T]"(w656) -> ()
        n383 = local write "T [K]"(w656) -> ()
        n384 = local write "Sweep Bias"(w656) -> ()
        n385 = local write "Fix Bias"(w656) -> ()
        n386 = local write "IOL ramp"(w656) -> ()
        n387 = local write "VI 4 Array"(w656) -> ()
      }
      frame "DACioload" {
        n388 = local read "DACindic"() -> (w661:bool)
        n389 = local read "DAC"() -> (w662:refnum<visa-resource-name>)
        n390 = case shown="True" w661 {
          tunnel: w662 -> [w664 w666]
          tunnel: "init" -> [w663 w665]
          tunnel: [w663 w665] -> w659
          frame False {
            n391 = call "closeRS232.vi"("VISA resource name"=w664) -> ()  [unwired: 2 in]
          }
          frame True {
            n392 = call "openRS232.vi"("com"=w666) -> ("VISA resource name"=w667:refnum<visa-resource-name>)  [unwired: 1 out]
            n393 = global write "Visa name1.vi" "VISA name"(w667) -> ()
          }
        }
      }
      frame "FCprocedure" {
        n394 = while {
          tunnel: "init" -> [w675]
          tunnel: [w675] -> w668
          shift-right: [w673] -> _
          shift-left: "setfield" -> [w676]
          tunnel: [FALSE] -> w669
          stop <- w674 stop-if-true
          n395 = case shown="\"gumsIT\"" w676 {
            tunnel: [TRUE _ _ _ _ _] -> w674
            tunnel: ["" w688 "wait" "RampField2Zero" w713 w730] -> w673
            frame "out", Default {
              n396 = global write "stopButton.vi" "stopsignal"(FALSE) -> ()
              n397 = local write "I am"("finished") -> ()
            }
            frame "setfield" {
              n398 = local read "counter 2"() -> (w682:i32)
              n399 = local read "Bipolar"() -> (w683:bool)
              n400 = local read "Cooling field (T)"() -> (w686:dbl)
              n401 = Greater Than 0?(x=w682) -> (x > 0?=w681:bool)
              n402 = local read "sweep rate B (T/min)"() -> (w691:dbl)
              n403 = local write "I am"("Ramping the field up") -> ()
              n404 = And(x=w683, y=w681) -> (x .and. y?=w684:bool)
              n405 = case shown="True" w684 {
                tunnel: [w694 w695] -> w685
                tunnel: w686 -> [w694 w697]
                frame False {
                }
                frame True {
                  n406 = Multiply(x=w697, y=-1.0) -> (x*y=w695:dbl)
                }
              }
              n407 = node(w691) -> (w690:dbl[unit])
              n408 = node(w685) -> (w692:dbl[unit])
              n409 = call "TeslSetField.vi"("Set Persistent"=TRUE, "Sweep rate"=w690, "Field required:"=w692) -> ("OK?"=w689:bool)  [unwired: 1 in, 1 out]
              n410 = case shown="False" w689 {
                selector: w689 -> [w699 w700]
                tunnel: ["out" "cooldown"] -> w688
                frame False {
                  n411 = local write "Field ok !"(w699) -> ()
                }
                frame True {
                  "Field ok !" <- w700
                }
              }
            }
            frame "cooldown" {
              n412 = local read "Base T (K)"() -> (w702:dbl)
              n413 = local read "ITC ref"() -> (w704:T1)
              n414 = call "Tloop.vi"("ITCSignal"=w704, "T target [K]"=w702, "Regulate ?"=TRUE) -> ()  [unwired: 2 in, 2 out]
              n415 = local write "I am"("Cooling down to base T") -> ()
            }
            frame "wait" {
              n416 = local write "I am"("Waiting") -> ()
              n417 = local read "Waiting time (min)"() -> (w709:dbl)
              n418 = Multiply(x=w709, y=60000.0) -> (x*y=w711:dbl)
              n419 = Wait (ms)(milliseconds to wait=w711) -> ()  [unwired: 1 out]
            }
            frame "RampField2Zero" {
              n420 = case shown="False" FALSE {
                tunnel: ["gumsIT" "degauss"] -> w713
                frame False {
                }
                frame True {
                  # "To be done"
                }
              }
              n421 = local read "sweep rate B (T/min)"() -> (w717:dbl)
              n422 = node(w717) -> (w718:dbl[unit])
              n423 = local write "I am"("Ramping the field back to zero") -> ()
              n424 = call "TeslSetField.vi"("Set Persistent"=TRUE, "Sweep rate"=w718, "Field required:"=dbl[unit] 0.0) -> ()  [unwired: 1 in, 2 out]
            }
            frame "gumsIT" {
              n425 = global write "stopButton.vi" "stopsignal"(FALSE) -> ()
              n426 = local read "Gain Cluster"() -> (w734:T4)
              n427 = local read "High T (K)"() -> (w728:dbl)
              n428 = local read "Base T (K)"() -> (w729:dbl)
              n429 = local read "counter 2"() -> (w725:i32)
              n430 = local read "Bipolar"() -> (w731:bool)
              n431 = local read "Refresh Rate [ms]"() -> (w732:i32)
              n432 = local read "Device Cluster"() -> (w733:T3)
              n433 = local read "File Basename"() -> (w738:string)
              n434 = local read "Folder Name"() -> (w737:path)
              n435 = local read "Temperature Up rate (K/min)"() -> (w727:dbl)
              n436 = call "autoNameFile.vi"("num"=w725, "File Basename"=w738, "Folder Name"=w737) -> ("path"=w736:path)
              n437 = call "gums_measureLoopV3.vi"("File Name"=w736, "SaveDataQuery"=TRUE, "Gain Cluster 2"=w734, "Refresh Rate [ms]"=w732, "Device Cluster"=w733) -> ()  [unwired: 6 in]
              n438 = local read "ITC ref"() -> (w726:T1)
              n439 = call "Tloop.vi"("ITCSignal"=w726, "T target [K]"=w729, "Precision"=w728, "Time limit"=w727) -> ("ITCSignal 2"=w724:T1, "Finish"=w723:bool)  [unwired: 1 in]
              n440 = local write "I am"("Heating up and acquiring hopefully amazing data") -> ()
              n441 = case shown="True" w731 {
                tunnel: w725 -> [_ w744]
                tunnel: ["out" w740] -> w730
                tunnel: w724 -> [_ _]
                frame False {
                }
                frame True {
                  n442 = Increment(x=w744) -> (x+1=w741:i32)
                  n443 = local write "counter 2"(w741) -> ()
                  n444 = Greater?(x=w741, y=1) -> (0:w743:bool)
                  n445 = case shown="True" w743 {
                    tunnel: w741 -> [w746 w748]
                    tunnel: [w746 w748] -> _
                    tunnel: ["setfield" "out"] -> w740
                    frame False {
                    }
                    frame True {
                    }
                  }
                }
              }
              n446 = global write "stopButton.vi" "stopsignal"(w723) -> ()
            }
          }
        }
        n447 = local write "START FC"(w669) -> ()
      }
      frame "PEMinit" {
        n448 = local read "PEM VISA"() -> (w749:refnum<visa-resource-name>)
        n449 = local read "PEM present ?"() -> (w751:bool)
        n450 = case shown="False" w751 {
          selector: w751 -> [w754 w756]
          tunnel: [w754 w756] -> w750
          tunnel: w749 -> [w753 w755]
          frame False {
            n451 = call "HindsPEM100_VISASeriaClose.vi"("VISA session (for class)"=w753) -> ()  [unwired: 18 in, 1 out]
          }
          frame True {
            n452 = call "HindsPEM100_VISA_Handle.vi"("VISA session"=w755) -> ("VISA refnum out"=w757:refnum<visa-resource-name>)  [unwired: 17 in, 1 out]
            n453 = global write "GlobalVar.vi" "PEM VISA"(w757) -> ()
          }
        }
        n454 = global write "GlobalVar.vi" "PEM present ?"(w750) -> ()
      }
      frame "setRetard" {
        n455 = local read "PEM present ?"() -> (w758:bool)
        n456 = case shown="True" w758 {
          frame False {
          }
          frame True {
            n457 = local read "PEM VISA"() -> (w760:refnum<visa-resource-name>)
            n458 = local read "PEM retardation (lambda)"() -> (w761:dbl)
            n459 = call "HindsPEM100_SetRetardation.vi"("VISA refnum in"=w760, "Retardation"=w761) -> ()  [unwired: 16 in, 2 out]
          }
        }
      }
    }
    "x .or. y?" <- w27
  }
  n460 = Unbundle By Name("Gain Cluster") -> ("conversion factor BG"=→"conversion factor sweep":dbl, "Vin / Vout 1"=→"Bias factor":dbl)  [unwired: 10 out]
  n461 = local write "Sweep Bias"(w9) -> ()
  n462 = Unbundle By Name("Device Cluster") -> ("K2400 1"=→"K2400 1":refnum<visa-resource-name>, "LockinX"=→"LockinX":string[][], "K2400 2"=→"K2400 2":refnum<visa-resource-name>, "DAC"=w6:refnum<visa-resource-name>, "ITC signal"=→"ITC ref":T1, "DAC present"=w7:bool, "DMMX"=→"DMMX":string[][])  [unwired: 3 out]
  "DAC" <- w6
  n463 = case shown="True" w7 {
    tunnel: w6 -> [_ w762]
    frame False {
    }
    frame True {
      n464 = call "openRS232.vi"("com"=w762) -> ("VISA resource name"=w763:refnum<visa-resource-name>)  [unwired: 1 out]
      n465 = global write "Visa name1.vi" "VISA name"(w763) -> ()
    }
  }
  "Nb Sweep Indicator" <- 1 ("Nb Sweep Indicator")
  "Nb Loop Indicator" <- 0.0 ("Nb Sweep Indicator")
